vi "HTRB Main.vi"() -> ()   [LabVIEW 2017]
uses:
  Controls/(Ctrl) System State.ctl
  Controls/(Ctrl) State_Test Manage.ctl
  <vilib>/Utility/miscctls.llb/LVPointTypeDef.ctl
  Controls/(Ctrl) State_Display Loop.ctl
  Controls/(Ctrl) State_HVPS CMD.ctl
  Controls/(Ctrl) State_Parcing.ctl
  Controls/(Ctrl) State_Chamber.ctl
  Variables/(Var) Get_HVPS_1.vi
  Variables/(Var) Get_HVPS_2.vi
  Variables/(Var) Get_HVPS_3.vi
  Variables/(Var) Chamber.vi
panel:
  out "G3. State":T1
  out "G2. State":T1
  out "G1. State":T1
  out "Pulse":bool
  out "END":bool=TRUE
  out "G3_TEST END?":bool
  out "G2_TEST END?":bool
  out "G1_TEST END?":bool
  out "Exit ?":bool
  out "탭 컨트롤":enum32{"Display", "Manual Mode", "State"}(tab)
  in  "Start Delay":dbl format="%<%H:%M:%S>t"
  out "G2. Operating Voltage":dbl caption="Operating Voltage" format="%.1f    V"
  in  "G2. Start Delay":dbl caption="Start Delay" format="%<%H:%M:%S>t"
  in  "G1. Start Delay":dbl caption="Start Delay" format="%<%H:%M:%S>t"
  in  "Group3. Info":string
  in  "Group2. Info":string
  in  "Group1. Info":string
  in  "Chamber":bool
  out "G3. Delay":dbl format="%<%H:%M:%S>t"
  out "G2. Delay":dbl format="%<%H:%M:%S>t"
  out "G1. Delay":dbl format="%<%H:%M:%S>t"
  out "G1. Current Graph":cluster{"G1. Current Limit ":dbl, "G1. mA":dbl}(graph)
  out "G1. Voltage Graph":dbl(graph)
  in  "Target Temp":u16 format="%d ℃"
  out "G3. Time":dbl format="%<%H:%M:%S>t"
  in  "G3. Target Time":dbl=460800.0 format="%<%H>t 시간"
  out "G2. Time":dbl format="%<%H:%M:%S>t"
  in  "G2. Target Time":dbl=460800.0 format="%<%H>t 시간"
  out "G1. Time":dbl format="%<%H:%M:%S>t"
  in  "G1. Target Time":dbl=460800.0 format="%<%H>t 시간"
  out "Chamber Temp":dbl format="%.2f ℃"
  out "G3. Current Graph":cluster{"G1. Current Limit ":dbl, "G1. mA":dbl}(graph)
  out "G3. Voltage Graph":dbl(graph)
  out "G2. Current Graph":cluster{"G1. Current Limit ":dbl, "G1. mA":dbl}(graph)
  out "G2. Voltage Graph":dbl(graph)
  in  "Data Save Path":path=path "D:/Raw"
  in  "G3. Stop Butten":bool
  in  "G3. Start Butten":bool
  in  "G2. Stop Butten":bool
  in  "G2. Start Butten":bool
  in  "G1. Stop Butten":bool
  in  "G1. Start Butten":bool
  in  "G2. Taget Voltage":dbl caption="Target Voltage" min=0.0 max=2000.0 format="%.1f V"
  in  "G1. Taget Voltage":dbl caption="Target Voltage" min=0.0 max=2000.0 format="%.1f V"
  in  "G3. Taget Voltage":dbl caption="Target Voltage" min=0.0 max=2000.0 format="%.1f V"
  in  "G3. RB/GB":bool
  out "G3. Test  Status":u16(ring)=1 caption="Test Status"
  out "G3.Comm":bool caption="Communication ="
  out "G3.System":bool caption="System Status ="
  out "G3. Operating Voltage":dbl caption="Operating Voltage" format="%.1f    V"
  out "G3. Leakage Current":dbl caption="Leakage Current" format="%.2f mA"
  in  "G3. Current Limit":dbl caption="Current Limit" format="%.1f mA"
  out "G3. Layout":bool
  in  "G2. RB/GB":bool
  out "G2. Test  Status":u16(ring)=1 caption="Test Status"
  out "G2.Comm":bool caption="Communication ="
  out "G2.System":bool caption="System Status ="
  out "G2. Leakage Current":dbl caption="Leakage Current" format="%.2f mA"
  in  "G2. Current Limit":dbl caption="Current Limit" format="%.1f mA"
  out "G2. Layout":bool
  in  "G1. RB/GB":bool
  out "G1.Comm":bool caption="Communication ="
  out "G1.System":bool caption="System Status ="
  out "G1. Test  Status":u16(ring)=1 caption="Test Status"
  out "G1. Operating Voltage":dbl caption="Operating Voltage" format="%.1f    V"
  out "G1. Leakage Current":dbl caption="Leakage Current" format="%.2f mA"
  in  "G1. Current Limit":dbl caption="Current Limit" format="%.1f mA"
  out "G1. Layout":bool
  out "G1_Disable":bool=TRUE
  out "G3_Disable":bool=TRUE
  out "G2_Disable":bool=TRUE
  out "Data Filename":path
  in  "Exit":bool
  out "G3.Manual_Get mA":dbl format="%3.1f mA"
  out "G3.Manual_Get V":dbl format="%.1f V"
  in  "Group.3 Manual":T2 {"Set mA" items=["0mA"=0, "5mA"=5, "10mA"=10, "15mA"=15, "20mA"=20, "50mA"=50, "70mA"=70, "100mA"=100, "150mA"=150]; "Set V" items=["0V"=0, "10V"=10, "100V"=100, "300V"=300, "500V"=500, "700V"=700, "1000V"=1000, "1500V"=1500]}
  out "G2.Manual_Get mA":dbl format="%3.1f mA"
  out "G2.Manual_Get V":dbl format="%.1f V"
  in  "Group.2 Manual":T2 {"Set mA" items=["0mA"=0, "5mA"=5, "10mA"=10, "15mA"=15, "20mA"=20, "50mA"=50, "70mA"=70, "100mA"=100, "150mA"=150]; "Set V" items=["0V"=0, "10V"=10, "100V"=100, "300V"=300, "500V"=500, "700V"=700, "1000V"=1000, "1500V"=1500]}
  out "G1.Manual_Get mA":dbl format="%3.1f mA"
  out "G1.Manual_Get V":dbl format="%.1f V"
  in  "Group.1 Manual":T2 {"Set mA" items=["0mA"=0, "5mA"=5, "10mA"=10, "15mA"=15, "20mA"=20, "50mA"=50, "70mA"=70, "100mA"=100, "150mA"=150]; "Set V" items=["0V"=0, "10V"=10, "100V"=100, "300V"=300, "500V"=500, "700V"=700, "1000V"=1000, "1500V"=1500]}
  out "G1 System State":T3
  out "G2 System State":T3
  out "G3 System State":T3
  out "error out":errorcluster
  in  "error in (no error)":errorcluster
  in  "Radio_TAB":enum32{"Home", "Manual Mode"}(radio)
  # "ON"
  # "OFF"
  # "High Temperature Reverse Bias Tester"
  # "Software Version 0.0.1"
  # "Group 1"
  # "/"
  # "Group 2"
  # "/"
  # "Group 3"
  # "/"
  # "Group.3 Manual"
  # "Group.2 Manual"
  # "Group.1 Manual"
  # "Group.1 System State"
  # "Voltage Mode On"
  # "Current Mode On"
  # "HV On"
  # "Regulator Error"
  # "Local Mode"
  # "System Fault"
  # "Adjustable Overload Fault"
  # "Over Temperature"
  # "Arc Fault"
  # "Over Power"
  # "Over Current"
  # "Over Voltage Fault"
  # "HV Inhibited"
  # "Interlock open"
  # "Group.2 System State"
  # "Voltage Mode On"
  # "Current Mode On"
  # "HV On"
  # "Regulator Error"
  # "Local Mode"
  # "System Fault"
  # "Adjustable Overload Fault"
  # "Over Temperature"
  # "Arc Fault"
  # "Over Power"
  # "Over Current"
  # "Over Voltage Fault"
  # "HV Inhibited"
  # "Interlock open"
  # "Group.3 System State"
  # "Voltage Mode On"
  # "Current Mode On"
  # "HV On"
  # "Regulator Error"
  # "Local Mode"
  # "System Fault"
  # "Adjustable Overload Fault"
  # "Over Temperature"
  # "Arc Fault"
  # "Over Power"
  # "Over Current"
  # "Over Voltage Fault"
  # "HV Inhibited"
  # "Interlock open"
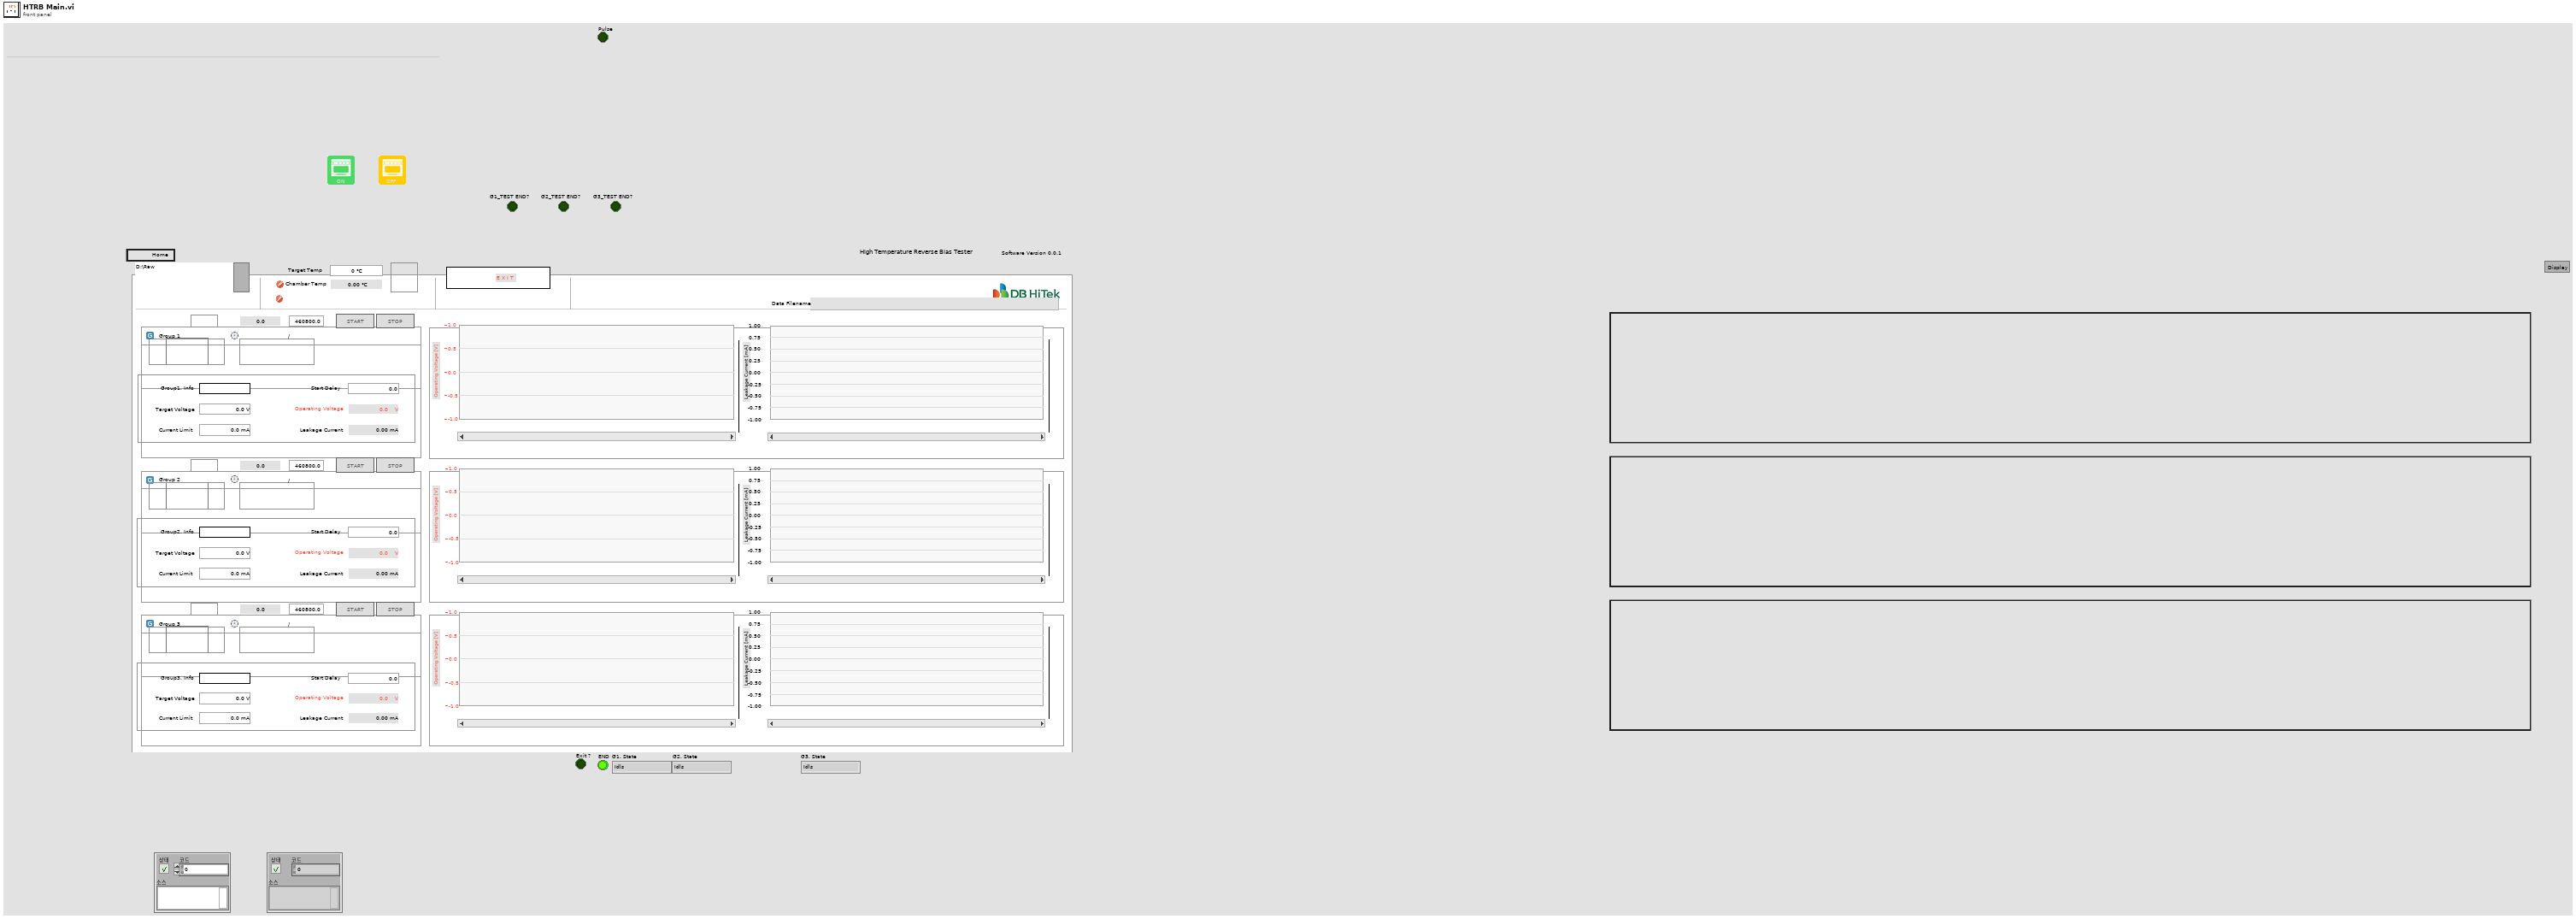
[diagram p1: front panel]
types:
  T1 = typedef "(Ctrl) State_Test Manage.ctl" = enum16{"Idls", "Run Init", "Run", "Rising", "Falling", "Quick Falling", "Close"}
  T2 = cluster{"Bool_HV ON":bool, "Bool_HV OFF":bool, "Bool_Set V":bool, "Bool_Set mA":bool, "Bool_Get V":bool, "Bool_Get mA":bool, "Set V":u16, "Set mA":u16}
  T3 = typedef "(Ctrl) System State.ctl" = cluster{"Interlock open":bool, "HV Inhibited":bool, "Over Voltage Fault":bool, "Over Current":bool, "Over Power":bool, "Regulator Error":bool, "Arc Fault":bool, "Over Temperature":bool, "Adjustable Overload Fault":bool, "System Fault":bool, "Remote Mode":bool, "HV On":bool, "Current Mode On":bool, "Voltage Mode On":bool}
  T4 = typedef "(Ctrl) State_Display Loop.ctl" = enum16{"Init", "Idls", "Run Init", "Run", "Stop", "Close"}
  T5 = typedef "LVPointTypeDef.ctl" = cluster{"Horizontal":i16, "Vertical":i16}
  T6 = typedef "(Ctrl) State_HVPS CMD.ctl" = enum16{"Open", "Rx : V", "Rx : mA", "Rx : State", "Rx : ADC", "Tx : Set V", "Tx : Set mA", "Tx : ON", "Tx : OFF", "Close"}
  T7 = enum8{"Enabled", "Disabled", "Disabled and Grayed Out"}
  T8 = typedef "(Ctrl) State_Chamber.ctl" = enum16{"Open", "Rx : Temp", "Rx : Target Temp", "Rx : State", "Tx : ON-OFF", "Tx : Target Temp", "Tx : Time Set", "Close"}
  T9 = enum16{"G1. Reset", "G2. Reset", "G3. Reset", "G1. Save", "G2. Save", "G3. Save", "G1. Load", "G2. Load", "G3. Load"}
  T10 = cluster{"G1. Current Limit ":dbl, "G1. mA":dbl}[]
  T11 = typedef "(Ctrl) State_Parcing.ctl" = enum16{"Default", "Set V", "Set mA", "Get V", "Get mA", "Get ADC"}
  T12 = enum32{"invalid app kind", "Development System", "Run Time System", "Student Edition", "Embedded LabVIEW", "Evaluation", "Custom"}
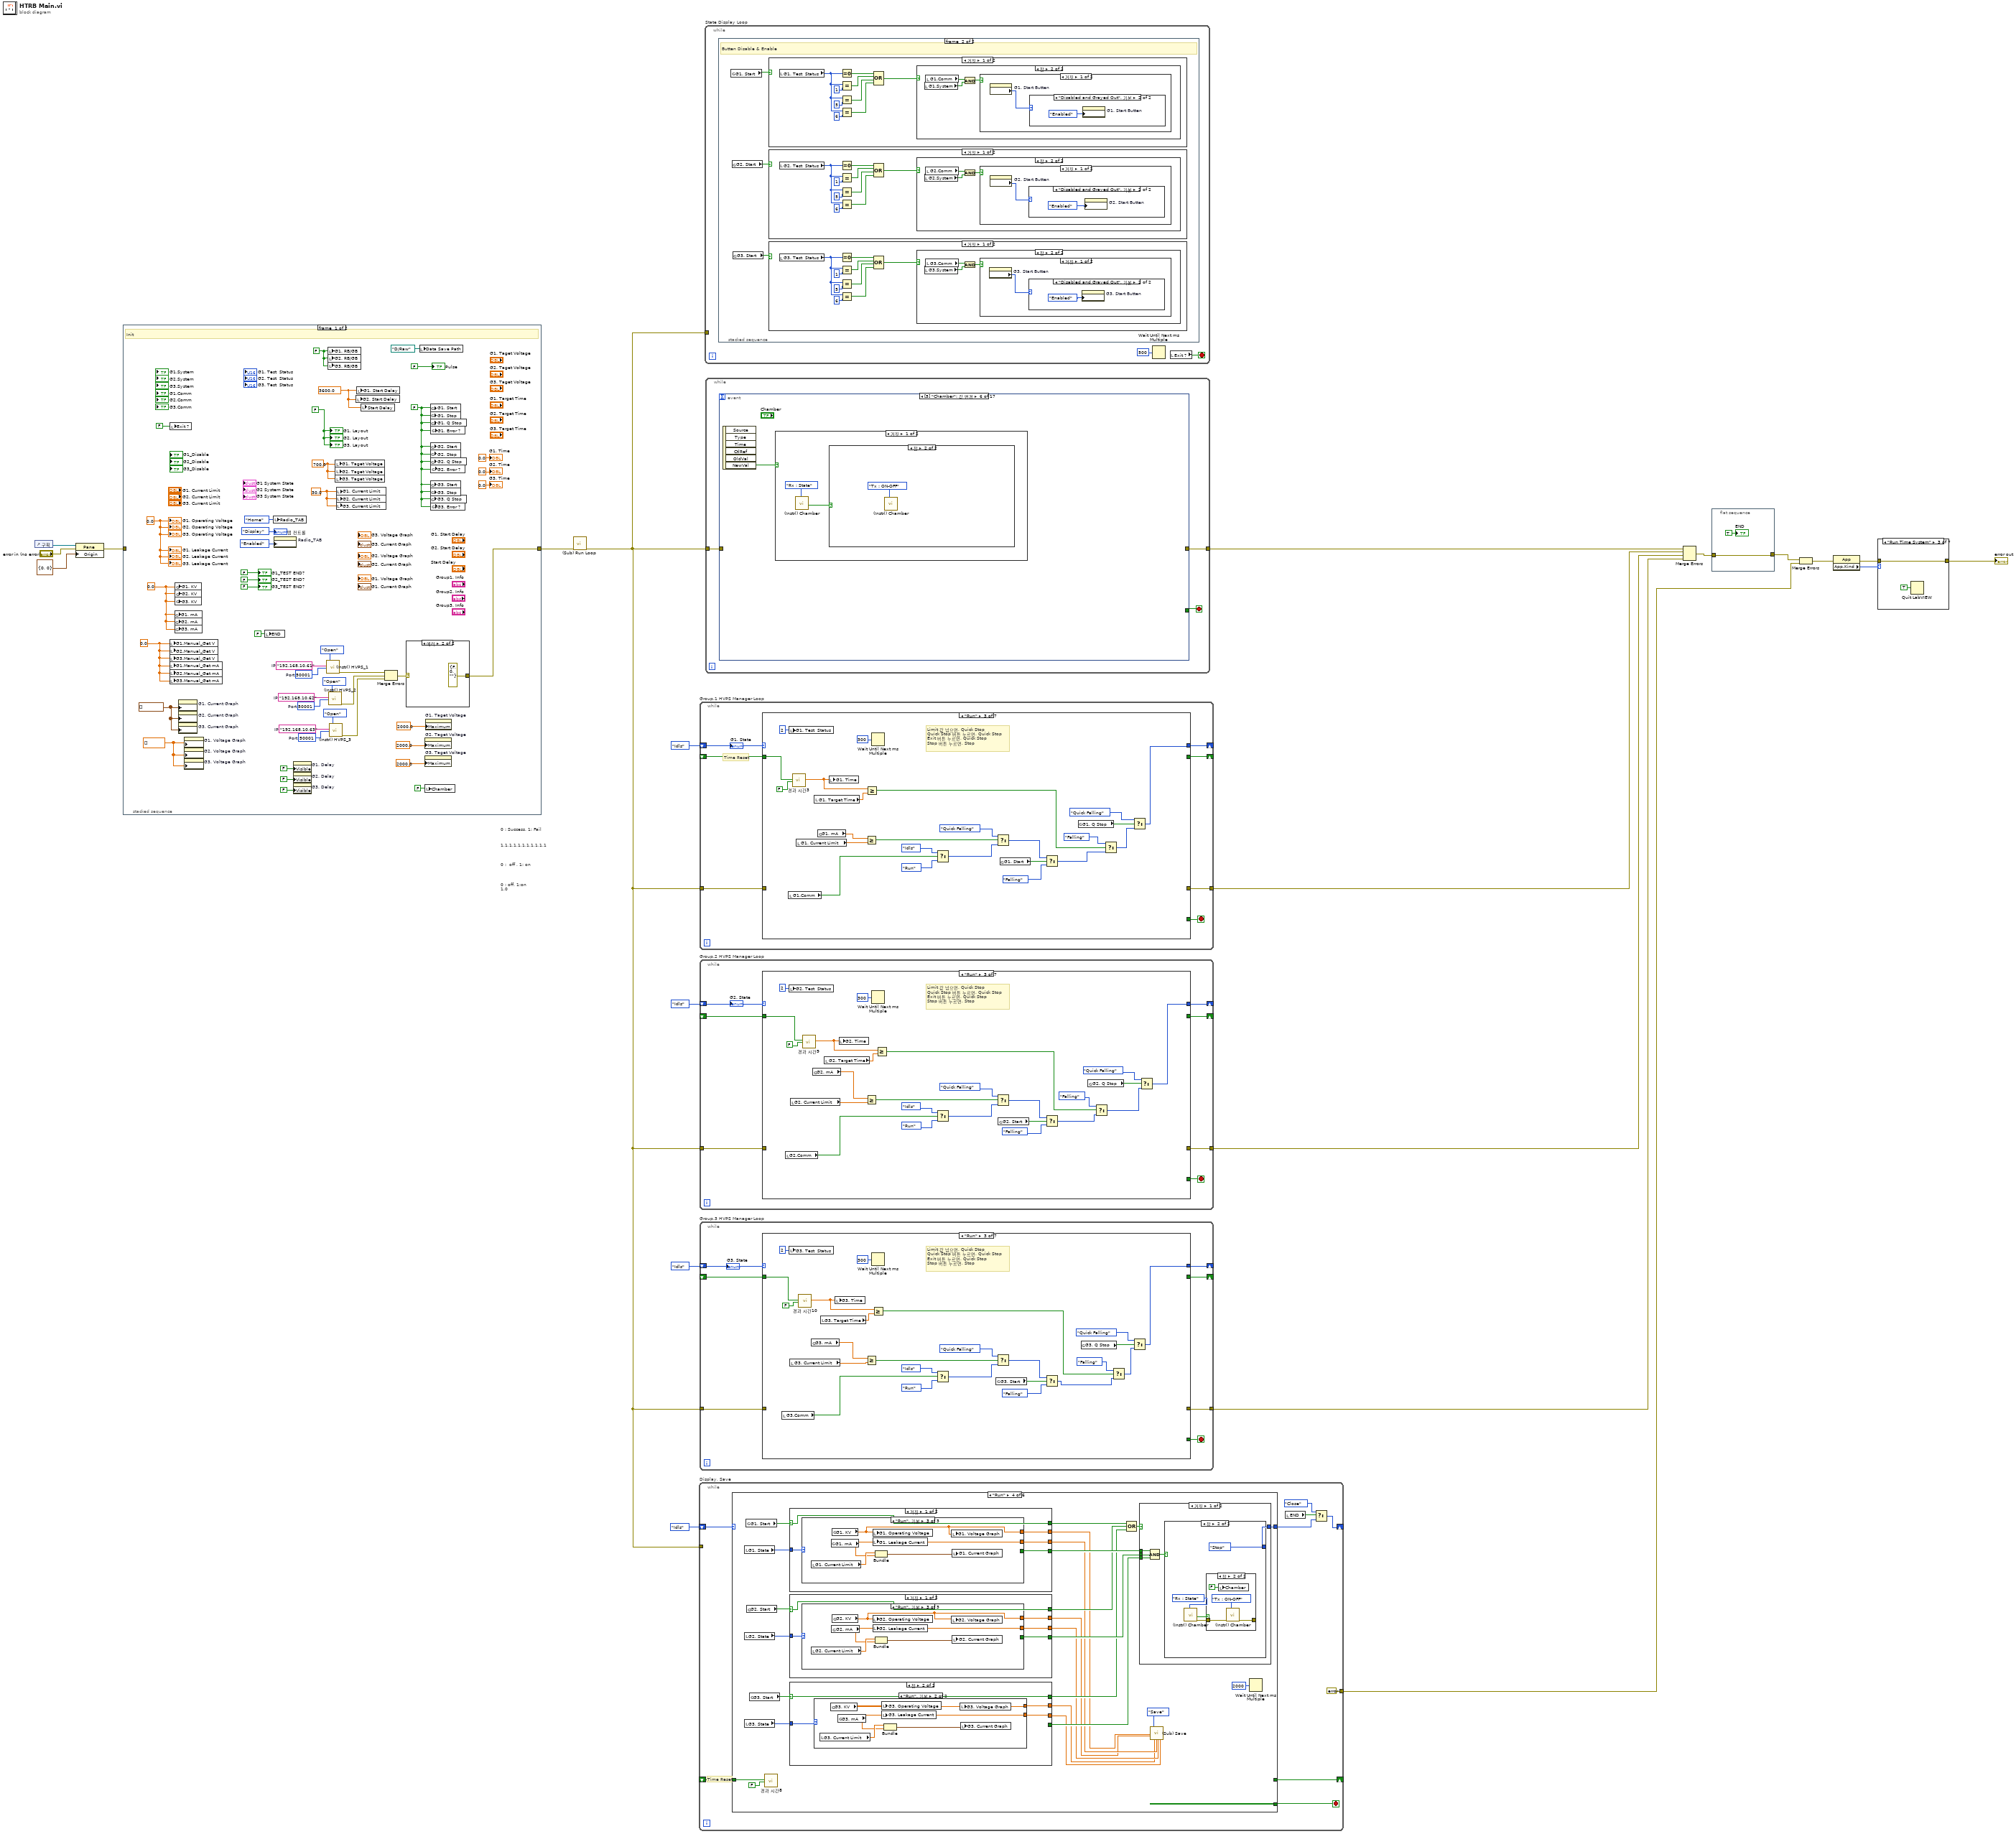
[diagram p0: block diagram]
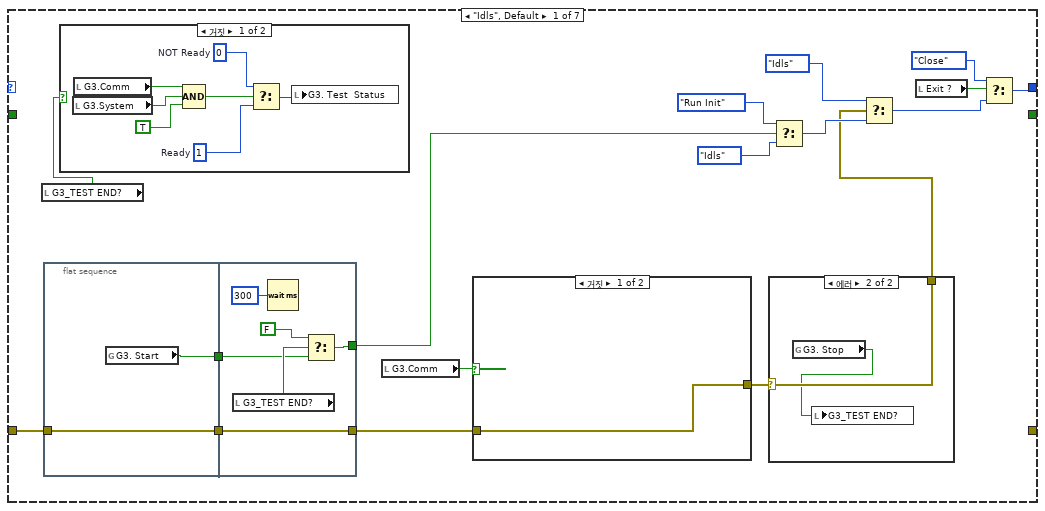
[diagram p2: hidden frame]
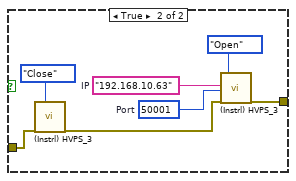
[diagram p3: hidden frame]
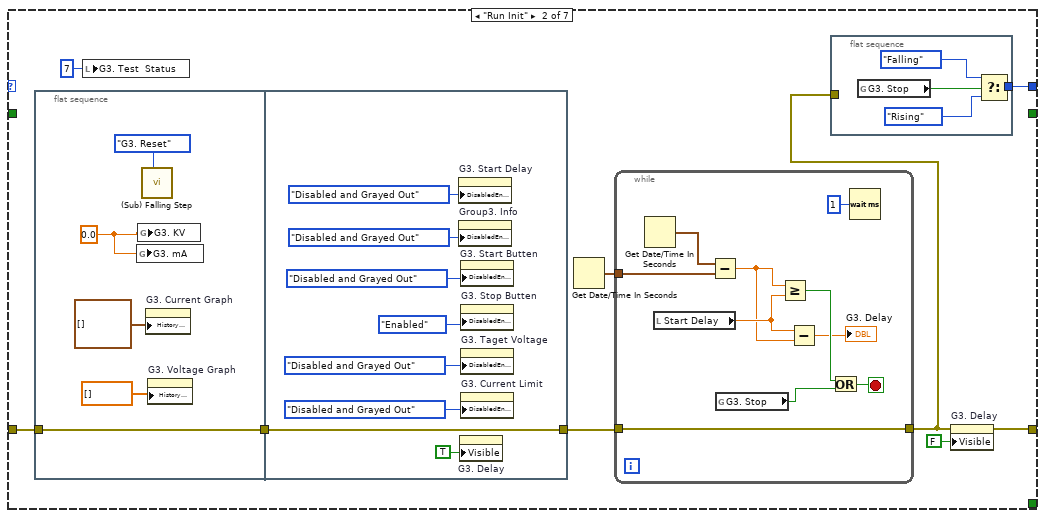
[diagram p6: hidden frame]
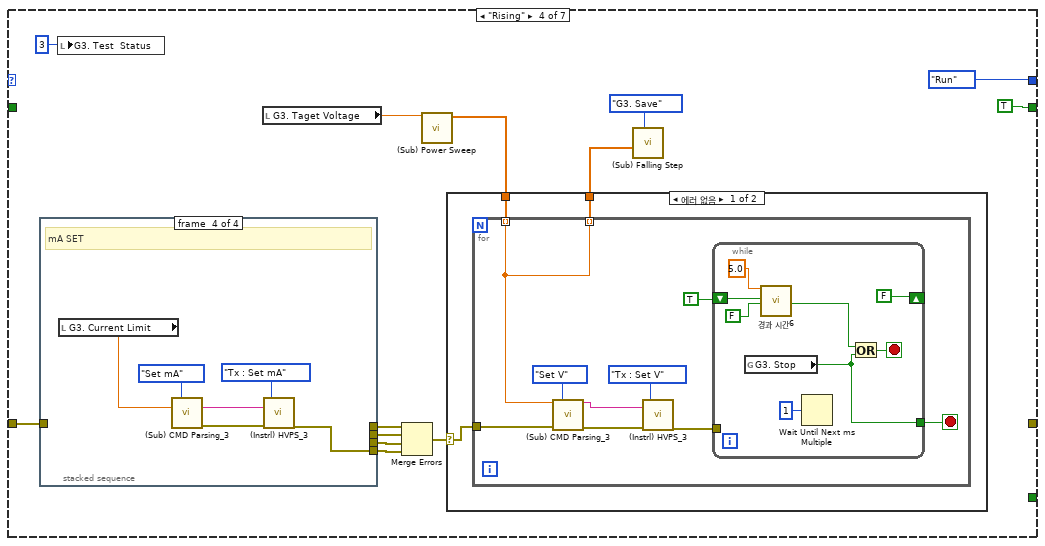
[diagram p7: hidden frame]
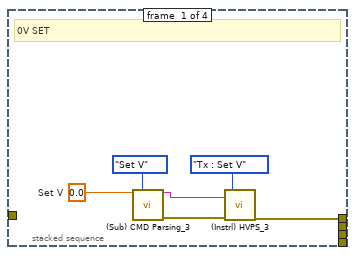
[diagram p9: hidden frame]
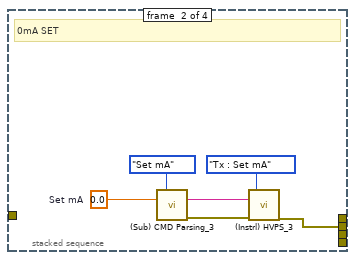
[diagram p10: hidden frame]
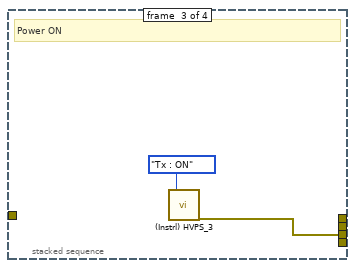
[diagram p11: hidden frame]
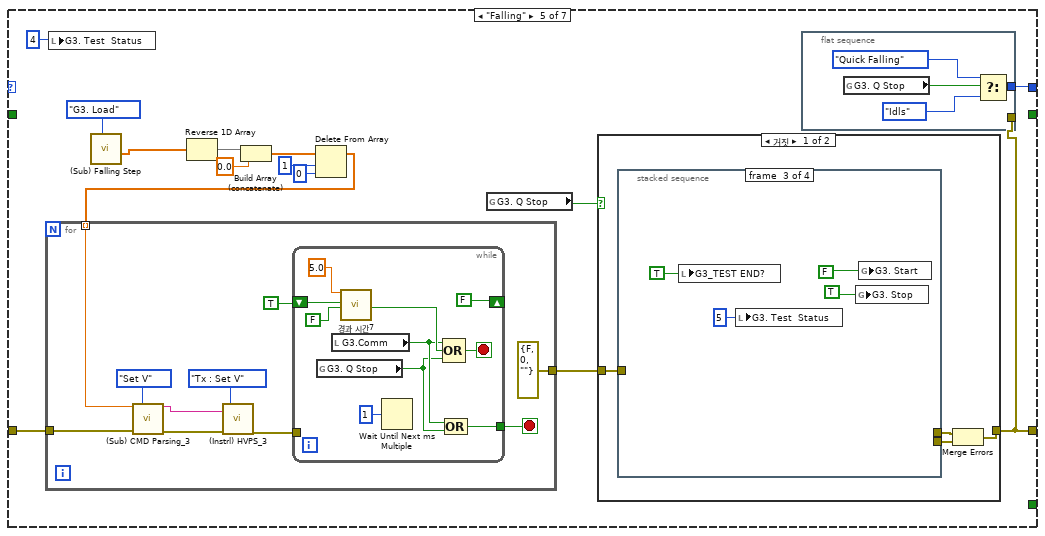
[diagram p12: hidden frame]
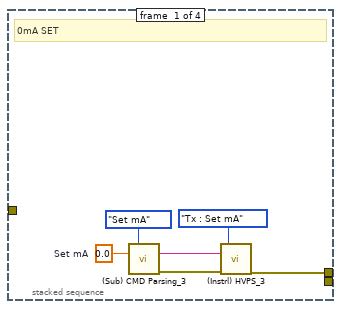
[diagram p13: hidden frame]
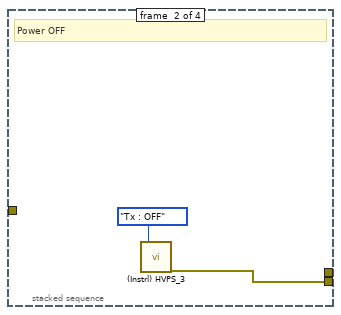
[diagram p14: hidden frame]
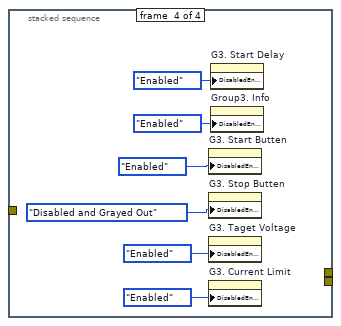
[diagram p15: hidden frame]
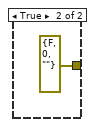
[diagram p16: hidden frame]
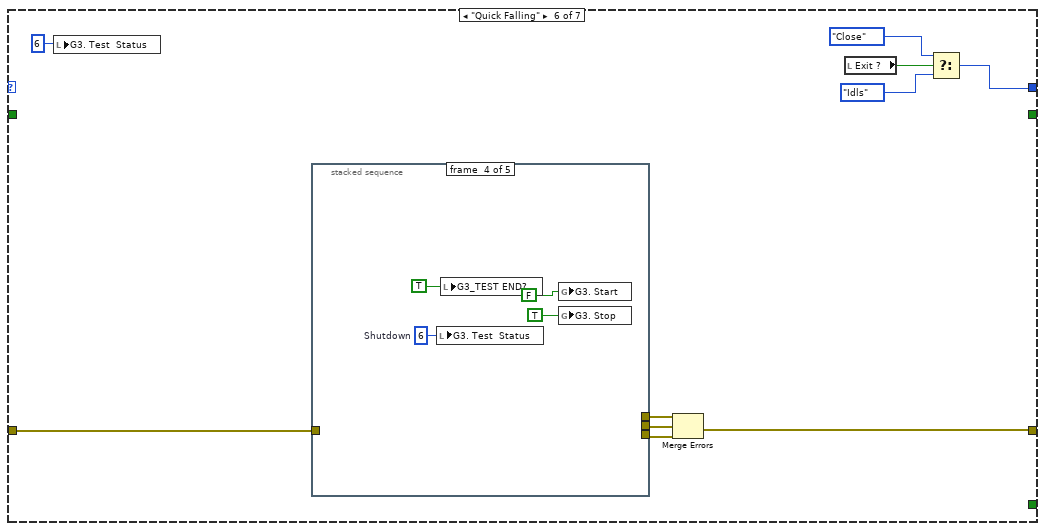
[diagram p17: hidden frame]
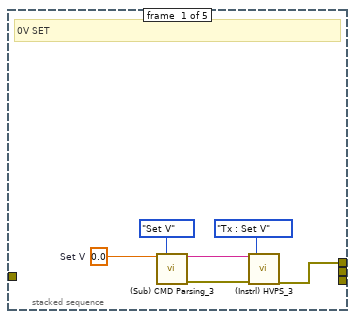
[diagram p18: hidden frame]
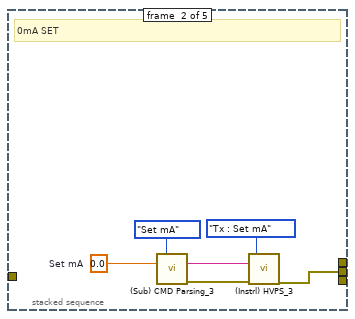
[diagram p19: hidden frame]
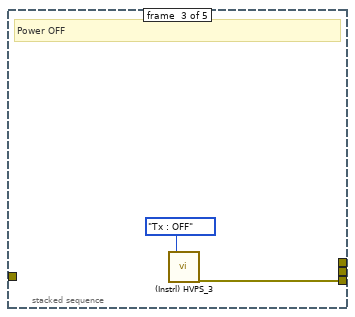
[diagram p20: hidden frame]
diagram:
  # "0 : off, 1:on\n1,0"
  # "0 :  off , 1: on"
  # "1,1,1,1,1,1,1,1,1,1,1"
  # "0 : Success, 1: Fail"
  n1 = control-ref of="구획"() -> (w15:refnum<vi>)
  n2 = property class="Pane"(reference=w15, error in="error in (no error)", "Origin"=T5 {"Horizontal"=0, "Vertical"=0} ("원점")) -> (error out=w12:errorcluster)  [unwired: 1 out]
  n3 = stacked-sequence {
    tunnel: w12 -> [_ _]
    tunnel: [w47 _] -> w2
    frame #0 {
      w27 = 3600.0
      w23 = FALSE
      w39 = FALSE
      w42 = 30.0
      w43 = 700.0
      w40 = FALSE
      w52 = u16 50001  # Port
      w53 = "192.168.10.63"  # IP
      w55 = u16 50001  # Port
      w56 = "192.168.10.62"  # IP
      w58 = u16 50001  # Port
      w59 = "192.168.10.61"  # IP
      w65 = 0.0 ("G1.Manual_Get V")
      w64 = 0.0 ("G1. Current Limit")
      w22 = 0.0 ("G1. KV")
      w38 = cluster{"Current Limit":dbl, "Current":dbl}[] [] ("히스토리 데이터")
      w37 = dbl[] [] ("히스토리 데이터")
      # "Init"
      n4 = local write "G1.Manual_Get V"(w65) -> ()
      n5 = local write "G2.Manual_Get V"(w65) -> ()
      n6 = local write "G3.Manual_Get V"(w65) -> ()
      n7 = local write "G1.Manual_Get mA"(w65) -> ()
      n8 = local write "G2.Manual_Get mA"(w65) -> ()
      n9 = local write "G3.Manual_Get mA"(w65) -> ()
      n10 = local write "Exit ?"(FALSE ("Exit ?")) -> ()
      n11 = global write "(Var) Get_HVPS_1.vi" "G1. mA"(w22) -> ()
      n12 = global write "(Var) Get_HVPS_2.vi" "G2. mA"(w22) -> ()
      n13 = global write "(Var) Get_HVPS_3.vi" "G3. mA"(w22) -> ()
      n14 = global write "(Var) Get_HVPS_1.vi" "G1. KV"(w22) -> ()
      n15 = global write "(Var) Get_HVPS_2.vi" "G2. KV"(w22) -> ()
      n16 = global write "(Var) Get_HVPS_3.vi" "G3. KV"(w22) -> ()
      n17 = property on="G1. Current Graph" class="WFChart (엄격한)"("History Data"=w38) -> ()  [unwired: 2 in, 2 out]
      n18 = property on="G2. Current Graph" class="WFChart (엄격한)"("History Data"=w38) -> ()  [unwired: 2 in, 2 out]
      n19 = property on="G3. Current Graph" class="WFChart (엄격한)"("History Data"=w38) -> ()  [unwired: 2 in, 2 out]
      n20 = property on="G1. Voltage Graph" class="WFChart (엄격한)"("History Data"=w37) -> ()  [unwired: 2 in, 2 out]
      n21 = property on="G2. Voltage Graph" class="WFChart (엄격한)"("History Data"=w37) -> ()  [unwired: 2 in, 2 out]
      n22 = property on="G3. Voltage Graph" class="WFChart (엄격한)"("History Data"=w37) -> ()  [unwired: 2 in, 2 out]
      n23 = local write "END"(FALSE ("END")) -> ()
      n24 = local write "Radio_TAB"(enum32{"Home", "Manual Mode"}."Home" ("Radio_TAB")) -> ()
      n25 = property on="Radio_TAB" class="RadioBtnsControl (엄격한)"("DisabledEnum"=T7."Enabled" ("비활성화")) -> ()  [unwired: 2 in, 2 out]
      n26 = property on="G1. Delay" class="DigNum (엄격한)"("Visible"=FALSE ("보이기")) -> ()  [unwired: 2 in, 2 out]
      n27 = property on="G2. Delay" class="DigNum (엄격한)"("Visible"=FALSE ("보이기")) -> ()  [unwired: 2 in, 2 out]
      n28 = property on="G3. Delay" class="DigNum (엄격한)"("Visible"=FALSE ("보이기")) -> ()  [unwired: 2 in, 2 out]
      n29 = call "(Instrl) HVPS_1.vi"("IP"=w59, "Port"=w58, "CMD"=(Ctrl)_State_HVPS_CMD."Open" ("State")) -> ("error out"=w51:errorcluster)  [unwired: 11 in, 5 out]
      n30 = local write "G1. RB/GB"(w40) -> ()
      n31 = local write "G2. RB/GB"(w40) -> ()
      n32 = local write "G3. RB/GB"(w40) -> ()
      n33 = call "(Instrl) HVPS_2.vi"("IP"=w56, "Port"=w55, "CMD"=(Ctrl)_State_HVPS_CMD."Open" ("State")) -> ("error out"=w50:errorcluster)  [unwired: 11 in, 5 out]
      n34 = call "(Instrl) HVPS_3.vi"("IP"=w53, "Port"=w52, "CMD"=(Ctrl)_State_HVPS_CMD."Open" ("State")) -> ("error out"=w49:errorcluster)  [unwired: 11 in, 5 out]
      n35 = local write "G1. Taget Voltage"(w43) -> ()
      n36 = local write "G2. Taget Voltage"(w43) -> ()
      n37 = local write "G3. Taget Voltage"(w43) -> ()
      n38 = local write "G1. Current Limit"(w42) -> ()
      n39 = local write "G2. Current Limit"(w42) -> ()
      n40 = local write "G3. Current Limit"(w42) -> ()
      n41 = local write "G2. Start Delay"(w27) -> ()
      n42 = local write "G1. Start Delay"(w27) -> ()
      n43 = local write "Start Delay"(w27) -> ()
      n44 = Merge Errors(w51, w50, w49) -> (w48:errorcluster)
      n45 = case shown="에러" w48 {
        selector: w48 -> [w67 _]
        tunnel: [w67 errorcluster {"status"=FALSE, "code"=0, "source"=""} ("에러 상수")] -> w47
        frame No Error {
        }
        frame Error {
        }
      }
      n46 = local write "Data Save Path"(path "D:/Raw" ("Data Save Path")) -> ()
      n47 = property on="G2. Taget Voltage" class="DigNum (엄격한)"("Maximum"=2000.0 ("데이터 입력 제한:최대")) -> ()  [unwired: 2 in, 2 out]
      n48 = property on="G3. Taget Voltage" class="DigNum (엄격한)"("Maximum"=2000.0 ("데이터 입력 제한:최대")) -> ()  [unwired: 2 in, 2 out]
      n49 = local write "Chamber"(FALSE ("Chamber")) -> ()
      n50 = property on="G1. Taget Voltage" class="DigNum (엄격한)"("Maximum"=2000.0 ("데이터 입력 제한:최대")) -> ()  [unwired: 2 in, 2 out]
      n51 = global write "(Var) Get_HVPS_1.vi" "G1. Start"(w23) -> ()
      n52 = global write "(Var) Get_HVPS_1.vi" "G1. Stop"(w23) -> ()
      n53 = global write "(Var) Get_HVPS_1.vi" "G1. Q Stop"(w23) -> ()
      n54 = global write "(Var) Get_HVPS_2.vi" "G2. Start"(w23) -> ()
      n55 = global write "(Var) Get_HVPS_2.vi" "G2. Stop"(w23) -> ()
      n56 = global write "(Var) Get_HVPS_2.vi" "G2. Q Stop"(w23) -> ()
      n57 = global write "(Var) Get_HVPS_3.vi" "G3. Start"(w23) -> ()
      n58 = global write "(Var) Get_HVPS_3.vi" "G3. Stop"(w23) -> ()
      n59 = global write "(Var) Get_HVPS_3.vi" "G3. Q Stop"(w23) -> ()
      n60 = global write "(Var) Get_HVPS_1.vi" "G1. Error ?"(w23) -> ()
      n61 = global write "(Var) Get_HVPS_2.vi" "G2. Error ?"(w23) -> ()
      n62 = global write "(Var) Get_HVPS_3.vi" "G3. Error ?"(w23) -> ()
      "G1. Leakage Current" <- w64
      "G1. Operating Voltage" <- w64
      "G2. Leakage Current" <- w64
      "G2. Operating Voltage" <- w64
      "G3. Leakage Current" <- w64
      "G3. Operating Voltage" <- w64
      "탭 컨트롤" <- enum32{"Display", "Manual Mode", "State"}."Display" ("탭 컨트롤")
      "G1_TEST END?" <- FALSE ("G1_TEST END?")
      "G2_TEST END?" <- FALSE ("G1_TEST END?")
      "G3_TEST END?" <- FALSE ("G1_TEST END?")
      "G1. Layout" <- w39
      "G3. Layout" <- w39
      "G2. Layout" <- w39
      "Pulse" <- FALSE
      "G1. Time" <- 0.0 ("G1. Time")
      "G2. Time" <- 0.0 ("G2. Time")
      "G3. Time" <- 0.0 ("G3. Time")
    }
    frame #1 {
      n63 = property on="G2. Start Delay" class="DigNum (엄격한)"("DisabledEnum"=T7."Enabled" ("비활성화")) -> ()  [unwired: 2 in, 2 out]
      n64 = property on="Group2. Info" class="Str"("DisabledEnum"=T7."Enabled" ("비활성화")) -> ()  [unwired: 2 in, 2 out]
      n65 = property on="G2. Start Butten" class="Bool"("DisabledEnum"=T7."Enabled" ("비활성화")) -> ()  [unwired: 2 in, 2 out]
      n66 = property on="G2. Stop Butten" class="Bool"("DisabledEnum"=T7."Disabled and Grayed Out" ("비활성화")) -> ()  [unwired: 2 in, 2 out]
      n67 = property on="G2. Taget Voltage" class="DigNum (엄격한)"("DisabledEnum"=T7."Enabled" ("비활성화")) -> ()  [unwired: 2 in, 2 out]
      n68 = property on="G2. Current Limit" class="DigNum (엄격한)"("DisabledEnum"=T7."Enabled" ("비활성화")) -> ()  [unwired: 2 in, 2 out]
      n69 = property on="G3. Start Butten" class="Bool"("DisabledEnum"=T7."Enabled" ("비활성화")) -> ()  [unwired: 2 in, 2 out]
      n70 = property on="G3. Stop Butten" class="Bool"("DisabledEnum"=T7."Disabled and Grayed Out" ("비활성화")) -> ()  [unwired: 2 in, 2 out]
      n71 = property on="G3. Taget Voltage" class="DigNum (엄격한)"("DisabledEnum"=T7."Enabled" ("비활성화")) -> ()  [unwired: 2 in, 2 out]
      n72 = property on="G3. Current Limit" class="DigNum (엄격한)"("DisabledEnum"=T7."Enabled" ("비활성화")) -> ()  [unwired: 2 in, 2 out]
      n73 = property on="G1. Start Butten" class="Bool"("DisabledEnum"=T7."Enabled" ("비활성화")) -> ()  [unwired: 2 in, 2 out]
      n74 = property on="G1. Stop Butten" class="Bool"("DisabledEnum"=T7."Disabled and Grayed Out" ("비활성화")) -> ()  [unwired: 2 in, 2 out]
      n75 = property on="G1. Taget Voltage" class="DigNum (엄격한)"("DisabledEnum"=T7."Enabled" ("비활성화")) -> ()  [unwired: 2 in, 2 out]
      n76 = property on="Group1. Info" class="Str"("DisabledEnum"=T7."Enabled" ("비활성화")) -> ()  [unwired: 2 in, 2 out]
      n77 = property on="Start Delay" class="DigNum (엄격한)"("DisabledEnum"=T7."Enabled" ("비활성화")) -> ()  [unwired: 2 in, 2 out]
      n78 = property on="G1. Start Delay" class="DigNum (엄격한)"("DisabledEnum"=T7."Enabled" ("비활성화")) -> ()  [unwired: 2 in, 2 out]
      n79 = property on="G1. Current Limit" class="DigNum (엄격한)"("DisabledEnum"=T7."Enabled" ("비활성화")) -> ()  [unwired: 2 in, 2 out]
      n80 = property on="Group3. Info" class="Str"("DisabledEnum"=T7."Enabled" ("비활성화")) -> ()  [unwired: 2 in, 2 out]
    }
  }
  n81 = call "(Sub) Run Loop.vi"("error in (no error)"=w2) -> ("error out"=w1:errorcluster)  [unwired: 10 in]
  n82 = while "Display, Save" {
    tunnel: w1 -> [_]
    tunnel: [errorcluster {"status"=FALSE, "code"=0, "source"=""} ("에러 상수")] -> w10
    shift-right: [w92] -> _
    shift-left: _ -> [w93]
    shift-right: [w90] -> _
    shift-left: (Ctrl)_State_Display_Loop."Idls" ("열거형") -> [w91]
    stop <- w95 stop-if-true
    # "Time Reset"
    n83 = case shown="\"Run\"" w91 {
      tunnel: [_ _ _ _ _ TRUE] -> w95
      tunnel: w93 -> [_ _ _ w150 _ _]
      tunnel: [TRUE _ TRUE _ _ _] -> w92
      tunnel: [_ w100 (Ctrl)_State_Display_Loop."Run" ("열거형") w148 (Ctrl)_State_Display_Loop."Idls" ("열거형") (Ctrl)_State_Display_Loop."Close" ("열거형")] -> w87
      frame "Init", Default {
      }
      frame "Idls" {
        n84 = Wait (ms)(milliseconds to wait=u32 300 ("ms 배수")) -> ()  [unwired: 1 out]
        n85 = global read "(Var) Get_HVPS_2.vi" "G2. Start"() -> (w98:bool)
        n86 = global read "(Var) Get_HVPS_3.vi" "G3. Start"() -> (w97:bool)
        n87 = global read "(Var) Get_HVPS_1.vi" "G1. Start"() -> (w99:bool)
        n88 = Compound Arithmetic op=OR ("복합 연산")(w99, w98, w97) -> (w103:bool)
        n89 = Select(t=(Ctrl)_State_Display_Loop."Run Init" ("열거형"), s=w103, f=(Ctrl)_State_Display_Loop."Idls" ("열거형")) -> (s? t:f=w100:T4)
      }
      frame "Run Init" {
        n90 = local read "G1. Taget Voltage"() -> (w111:dbl)
        n91 = local read "G2. Taget Voltage"() -> (w110:dbl)
        n92 = local read "G3. Taget Voltage"() -> (w109:dbl)
        n93 = local read "G1. Current Limit"() -> (w114:dbl)
        n94 = local read "G2. Current Limit"() -> (w113:dbl)
        n95 = local read "G3. Current Limit"() -> (w112:dbl)
        n96 = local read "Group1. Info"() -> (w107:string)
        n97 = local read "Group2. Info"() -> (w106:string)
        n98 = local read "Group3. Info"() -> (w105:string)
        n99 = Build Array(w114, w113, w112, w111, w110, w109) -> (w108:dbl[])
        n100 = flat-sequence {
          tunnel: "Data Save Path" -> [w122]
          tunnel: w108 -> [w120]
          tunnel: [w121] -> w117
          tunnel: [w120] -> w116
          tunnel: w107 -> [_]
          tunnel: w106 -> [_]
          tunnel: w105 -> [_]
          tunnel: w117 -> [w126]
          tunnel: w116 -> [w125]
          frame #0 {
            n101 = call "(Sub) Save.vi"("IN Path"=w122, "State"=enum16{"Open", "Header Make", "Save", "Close"}."Open") -> ("Save Path"=→"Data Filename":path, "error out"=w121:errorcluster)  [unwired: 16 in]
          }
          frame #1 {
            n102 = call "(Sub) Save.vi"("C Limit / Voltage"=w125, "error in (no error)"=w126, "State"=enum16{"Open", "Header Make", "Save", "Close"}."Header Make") -> ()  [unwired: 15 in, 2 out]
          }
        }
      }
      frame "Run" {
        n103 = local read "G1. State"() -> (w145:T1)
        n104 = local read "G2. State"() -> (w143:T1)
        n105 = local read "G3. State"() -> (w142:T1)
        n106 = global read "(Var) Get_HVPS_1.vi" "G1. Start"() -> (w137:bool)
        n107 = global read "(Var) Get_HVPS_2.vi" "G2. Start"() -> (w136:bool)
        n108 = global read "(Var) Get_HVPS_3.vi" "G3. Start"() -> (w135:bool)
        n109 = call "경과 시간8"("Reset"=w150, "Auto Reset"=FALSE) -> ()  [unwired: 10 in, 8 out]
        n110 = case shown="거짓" w137 {
          selector: w137 -> [w220 w236]
          tunnel: [w222 w235] -> w133
          tunnel: [w221 w234] -> w132
          tunnel: [w220 w236] -> w147
          tunnel: w145 -> [w219 w233]
          tunnel: [w218 _] -> w144
          frame False {
            n111 = case shown="\"Run\", 기본" w219 {
              tunnel: [nan nan w229] -> w222
              tunnel: [nan nan w230] -> w221
              tunnel: [TRUE TRUE _] -> w218
              frame "Idls" {
              }
              frame "Run Init" {
              }
              frame "Run", Default {
                n112 = local read "G1. Current Limit"() -> (w232:dbl)
                n113 = global read "(Var) Get_HVPS_1.vi" "G1. mA"() -> (w230:dbl)
                n114 = global read "(Var) Get_HVPS_1.vi" "G1. KV"() -> (w229:dbl)
                n115 = local write "G1. Operating Voltage"(w229) -> ()
                n116 = local write "G1. Leakage Current"(w230) -> ()
                n117 = Bundle("G1. Current Limit"=w232, "G1. mA"=w230) -> (w231:cluster{"G1. Current Limit ":dbl, "G1. mA":dbl})  [unwired: 1 in]
                n118 = local write "G1. Voltage Graph"(w229) -> ()
                n119 = local write "G1. Current Graph"(w231) -> ()
              }
            }
          }
          frame True {
            n120 = case shown="\"Run\", 기본" w233 {
              tunnel: [nan w240] -> w235
              tunnel: [nan w239] -> w234
              frame "Run Init" {
              }
              frame "Run", Default {
                n121 = local read "G1. Current Limit"() -> (w242:dbl)
                n122 = global read "(Var) Get_HVPS_1.vi" "G1. mA"() -> (w239:dbl)
                n123 = global read "(Var) Get_HVPS_1.vi" "G1. KV"() -> (w240:dbl)
                n124 = local write "G1. Operating Voltage"(w240) -> ()
                n125 = local write "G1. Leakage Current"(w239) -> ()
                n126 = Bundle("G1. Current Limit"=w242, "G1. mA"=w239) -> (w241:cluster{"G1. Current Limit ":dbl, "G1. mA":dbl})  [unwired: 1 in]
                n127 = local write "G1. Voltage Graph"(w240) -> ()
                n128 = local write "G1. Current Graph"(w241) -> ()
              }
            }
          }
        }
        n129 = case shown="거짓" w136 {
          selector: w136 -> [w179 w195]
          tunnel: [w181 w194] -> w131
          tunnel: [w180 w193] -> w130
          tunnel: [w179 w195] -> w141
          tunnel: w143 -> [w178 w192]
          tunnel: [w177 _] -> w140
          frame False {
            n130 = case shown="\"Run\", 기본" w178 {
              tunnel: [nan nan w188] -> w181
              tunnel: [nan nan w189] -> w180
              tunnel: [TRUE TRUE _] -> w177
              frame "Idls" {
              }
              frame "Run Init" {
              }
              frame "Run", Default {
                n131 = local read "G2. Current Limit"() -> (w191:dbl)
                n132 = global read "(Var) Get_HVPS_2.vi" "G2. mA"() -> (w189:dbl)
                n133 = global read "(Var) Get_HVPS_2.vi" "G2. KV"() -> (w188:dbl)
                n134 = local write "G2. Operating Voltage"(w188) -> ()
                n135 = local write "G2. Leakage Current"(w189) -> ()
                n136 = Bundle("G2. Current Limit"=w191, "G2. mA"=w189) -> (w190:cluster{"G2. Current Limit ":dbl, "G2. mA":dbl})  [unwired: 1 in]
                n137 = local write "G2. Voltage Graph"(w188) -> ()
                n138 = local write "G2. Current Graph"(w190) -> ()
              }
            }
          }
          frame True {
            n139 = case shown="\"Run\", 기본" w192 {
              tunnel: [nan w198] -> w194
              tunnel: [nan w199] -> w193
              frame "Run Init" {
              }
              frame "Run", Default {
                n140 = local read "G2. Current Limit"() -> (w201:dbl)
                n141 = global read "(Var) Get_HVPS_2.vi" "G2. mA"() -> (w199:dbl)
                n142 = global read "(Var) Get_HVPS_2.vi" "G2. KV"() -> (w198:dbl)
                n143 = local write "G2. Operating Voltage"(w198) -> ()
                n144 = local write "G2. Leakage Current"(w199) -> ()
                n145 = Bundle("G2. Current Limit"=w201, "G2. mA"=w199) -> (w200:cluster{"G2. Current Limit ":dbl, "G2. mA":dbl})  [unwired: 1 in]
                n146 = local write "G2. Voltage Graph"(w198) -> ()
                n147 = local write "G2. Current Graph"(w200) -> ()
              }
            }
          }
        }
        n148 = case shown="참" w135 {
          selector: w135 -> [w154 w170]
          tunnel: [w156 w169] -> w129
          tunnel: [w155 w168] -> w128
          tunnel: [w154 w170] -> w139
          tunnel: w142 -> [w153 w167]
          tunnel: [w152 _] -> w138
          frame False {
            n149 = case shown="\"Run\", 기본" w153 {
              tunnel: [nan nan w164] -> w156
              tunnel: [nan nan w163] -> w155
              tunnel: [TRUE TRUE _] -> w152
              frame "Idls" {
              }
              frame "Run Init" {
              }
              frame "Run", Default {
                n150 = local read "G3. Current Limit"() -> (w166:dbl)
                n151 = global read "(Var) Get_HVPS_3.vi" "G3. mA"() -> (w163:dbl)
                n152 = global read "(Var) Get_HVPS_3.vi" "G3. KV"() -> (w164:dbl)
                n153 = local write "G3. Operating Voltage"(w164) -> ()
                n154 = local write "G3. Leakage Current"(w163) -> ()
                n155 = Bundle("G3. Current Limit"=w166, "G3. mA"=w163) -> (w165:cluster{"G3. Current Limit ":dbl, "G3. mA":dbl})  [unwired: 1 in]
                n156 = local write "G3. Voltage Graph"(w164) -> ()
                n157 = local write "G3. Current Graph"(w165) -> ()
              }
            }
          }
          frame True {
            n158 = case shown="\"Run\", 기본" w167 {
              tunnel: [nan w174] -> w169
              tunnel: [nan w173] -> w168
              frame "Run Init" {
              }
              frame "Run", Default {
                n159 = local read "G3. Current Limit"() -> (w176:dbl)
                n160 = global read "(Var) Get_HVPS_3.vi" "G3. KV"() -> (w174:dbl)
                n161 = global read "(Var) Get_HVPS_3.vi" "G3. mA"() -> (w173:dbl)
                n162 = local write "G3. Operating Voltage"(w174) -> ()
                n163 = local write "G3. Leakage Current"(w173) -> ()
                n164 = Bundle("G3. Current Limit"=w176, "G3. mA"=w173) -> (w175:cluster{"G3. Current Limit ":dbl, "G3. mA":dbl})  [unwired: 1 in]
                n165 = local write "G3. Voltage Graph"(w174) -> ()
                n166 = local write "G3. Current Graph"(w175) -> ()
              }
            }
          }
        }
        n167 = Compound Arithmetic op=OR ("복합 연산")(w147, w141, w139) -> (w146:bool)
        n168 = case shown="거짓" w146 {
          tunnel: [w206 (Ctrl)_State_Display_Loop."Run" ("열거형")] -> w148
          tunnel: w144 -> [w205 _]
          tunnel: w140 -> [w204 _]
          tunnel: w138 -> [w203 _]
          frame False {
            n169 = Compound Arithmetic op=AND ("복합 연산")(w205, w204, w203) -> (w202:bool)
            n170 = case shown="참" w202 {
              tunnel: [(Ctrl)_State_Display_Loop."Run" ("열거형") (Ctrl)_State_Display_Loop."Stop" ("열거형")] -> w206
              frame False {
              }
              frame True {
                n171 = call "(Instrl) Chamber.vi"("State"=(Ctrl)_State_Chamber."Rx : State") -> ("error out"=w209:errorcluster, "Run ?"=w210:bool)  [unwired: 7 in, 2 out]
                n172 = case shown="참" w210 {
                  tunnel: w209 -> [w212 w216]
                  tunnel: [w212 w214] -> _
                  frame False {
                  }
                  frame True {
                    n173 = local write "Chamber"(FALSE ("Chamber")) -> ()
                    n174 = call "(Instrl) Chamber.vi"("State"=(Ctrl)_State_Chamber."Tx : ON-OFF", "error in (no error)"=w216) -> ("error out"=w214:errorcluster)  [unwired: 6 in, 3 out]
                  }
                }
              }
            }
          }
          frame True {
          }
        }
        n175 = call "(Sub) Save.vi"("G1. V"=w133, "G2. V"=w131, "State"=enum16{"Open", "Header Make", "Save", "Close"}."Save", "G3. V"=w129, "G1. A"=w132, "G2. A"=w130, "G3. A"=w128) -> ()  [unwired: 11 in, 2 out]
        n176 = Wait Until Next ms Multiple(millisecond multiple=u32 2000 ("대기 시간 (ms)")) -> ()  [unwired: 1 out]
      }
      frame "Stop" {
        n177 = property on="Pulse" class="Bool (엄격한)"("Val(Sgnl)"=FALSE ("값(신호)")) -> ()  [unwired: 2 in, 2 out]
      }
      frame "Close" {
      }
    }
    n178 = local read "END"() -> (w89:bool)
    n179 = Select(t=(Ctrl)_State_Display_Loop."Close" ("열거형"), s=w89, f=w87) -> (s? t:f=w90:T4)
  }
  n180 = while "Group.1 HVPS Manager Loop" {
    shift-right: [w252] -> _
    shift-left: (Ctrl)_State_Test_Manage."Idls" ("State") -> [w253]
    tunnel: w1 -> [w249]
    tunnel: [w250] -> w17
    shift-right: [w248] -> _
    shift-left: _ -> [w247]
    stop <- w251 stop-if-true
    # "Time Reset"
    n181 = case shown="\"Run\"" w253 {
      tunnel: [w263 w300 w346 (Ctrl)_State_Test_Manage."Run" ("State") w423 w480 (Ctrl)_State_Test_Manage."Close" ("State")] -> w252
      tunnel: [_ _ _ _ _ _ TRUE] -> w251
      tunnel: w249 -> [w267 w305 _ w369 w425 w482 w507]
      tunnel: [_ w298 _ _ w415 w474 w508] -> w250
      tunnel: [_ _ _ TRUE _ _ _] -> w248
      tunnel: w247 -> [_ _ w342 _ _ _ _]
      frame "Idls", Default {
        n182 = flat-sequence {
          tunnel: w267 -> [w290]
          tunnel: [w289] -> w269
          tunnel: [w290] -> w268
          tunnel: [w296] -> w262
          tunnel: w269 -> [w293]
          tunnel: w268 -> [w296]
          tunnel: [w291] -> w261
          frame #0 {
            n183 = global read "(Var) Get_HVPS_1.vi" "G1. Start"() -> (w289:bool)
          }
          frame #1 {
            n184 = local read "G1_TEST END?"() -> (w294:bool)
            n185 = Wait (ms)(milliseconds to wait=u32 300 ("대기 시간 (ms)")) -> ()  [unwired: 1 out]
            n186 = Select(t=FALSE, s=w294, f=w293) -> (s? t:f=w291:bool)
          }
        }
        n187 = local read "G1_TEST END?"() -> (w256:bool)
        n188 = case shown="거짓" w256 {
          frame False {
            w283 = 1  # Ready
            w284 = 0  # NOT Ready
            n189 = local read "G1.System"() -> (w287:bool)
            n190 = local read "G1.Comm"() -> (w288:bool)
            n191 = Compound Arithmetic op=AND(w288, w287, TRUE) -> (w285:bool)
            n192 = Select(t=w284, s=w285, f=w283) -> (s? t:f=w282:i32)
            n193 = local write "G1. Test  Status"(w282) -> ()
          }
          frame True {
          }
        }
        n194 = local read "G1.Comm"() -> (w254:bool)
        n195 = case shown="참" w254 {
          tunnel: w262 -> [w271 w274]
          tunnel: [w271 w277] -> w255
          frame False {
          }
          frame True {
            w275 = u16 50001  # Port
            w276 = "192.168.10.61"  # IP
            n196 = call "(Instrl) HVPS_1.vi"("error in (no error)"=w274, "CMD"=(Ctrl)_State_HVPS_CMD."Close" ("State")) -> ("error out"=w272:errorcluster)  [unwired: 12 in, 5 out]
            n197 = call "(Instrl) HVPS_1.vi"("IP"=w276, "Port"=w275, "error in (no error)"=w272, "CMD"=(Ctrl)_State_HVPS_CMD."Open" ("State")) -> ("error out"=w277:errorcluster)  [unwired: 10 in, 5 out]
          }
        }
        n198 = case shown="에러" w255 {
          selector: w255 -> [w279 w281]
          tunnel: [w279 w281] -> w258
          frame No Error {
          }
          frame Error {
            n199 = global read "(Var) Get_HVPS_1.vi" "G1. Stop"() -> (w280:bool)
            n200 = local write "G1_TEST END?"(w280) -> ()
          }
        }
        n201 = Select(t=(Ctrl)_State_Test_Manage."Run Init" ("State"), s=w261, f=(Ctrl)_State_Test_Manage."Idls" ("State")) -> (s? t:f=w260:T1)
        n202 = Select(t=(Ctrl)_State_Test_Manage."Idls" ("State"), s=w258, f=w260) -> (s? t:f=w257:T1)
        n203 = local read "Exit ?"() -> (w266:bool)
        n204 = Select(t=(Ctrl)_State_Test_Manage."Close" ("State"), s=w266, f=w257) -> (s? t:f=w263:T1)
      }
      frame "Run Init" {
        n205 = flat-sequence {
          tunnel: w305 -> [w324]
          tunnel: [w324] -> w304
          tunnel: [w332] -> w303
          tunnel: w304 -> [w332]
          frame #0 {
            w321 = 0.0 ("G1. KV")
            n206 = global write "(Var) Get_HVPS_1.vi" "G1. mA"(w321) -> ()
            n207 = global write "(Var) Get_HVPS_1.vi" "G1. KV"(w321) -> ()
            n208 = call "(Sub) Falling Step.vi"("State"=T9."G1. Reset") -> ()  [unwired: 7 in, 4 out]
            n209 = property on="G1. Voltage Graph" class="WFChart (엄격한)"("History Data"=dbl[] [] ("히스토리 데이터")) -> ()  [unwired: 2 in, 2 out]
            n210 = property on="G1. Current Graph" class="WFChart (엄격한)"("History Data"=T10 [] ("히스토리 데이터")) -> ()  [unwired: 2 in, 2 out]
          }
          frame #1 {
            n211 = property on="G1. Start Butten" class="Bool"("DisabledEnum"=T7."Disabled and Grayed Out" ("비활성화")) -> ()  [unwired: 2 in, 2 out]
            n212 = property on="G1. Stop Butten" class="Bool"("DisabledEnum"=T7."Enabled" ("비활성화")) -> ()  [unwired: 2 in, 2 out]
            n213 = property on="G1. Taget Voltage" class="DigNum (엄격한)"("DisabledEnum"=T7."Disabled and Grayed Out" ("비활성화")) -> ()  [unwired: 2 in, 2 out]
            n214 = property on="Group1. Info" class="Str"("DisabledEnum"=T7."Disabled and Grayed Out" ("비활성화")) -> ()  [unwired: 2 in, 2 out]
            n215 = property on="G1. Current Limit" class="DigNum (엄격한)"("DisabledEnum"=T7."Disabled and Grayed Out" ("비활성화")) -> ()  [unwired: 2 in, 2 out]
            n216 = property on="G1. Start Delay" class="DigNum (엄격한)"("DisabledEnum"=T7."Disabled and Grayed Out" ("비활성화")) -> ()  [unwired: 2 in, 2 out]
            n217 = property on="G1. Delay" class="DigNum (엄격한)"("Visible"=TRUE ("보이기")) -> ()  [unwired: 2 in, 2 out]
          }
        }
        n218 = local write "G1. Test  Status"(u16 7 ("G1. Test  Status")) -> ()
        n219 = Get Date/Time In Seconds() -> (seconds since 1Jan1904=w302:timestamp)
        n220 = while {
          tunnel: w303 -> [w319]
          tunnel: [w319] -> w297
          tunnel: w302 -> [w318]
          stop <- w314 stop-if-true
          n221 = local read "G1. Start Delay"() -> (w313:dbl)
          n222 = Get Date/Time In Seconds() -> (seconds since 1Jan1904=w317:timestamp)
          n223 = Subtract(x=w317, y=w318) -> (x-y=w312:dbl)
          n224 = global read "(Var) Get_HVPS_1.vi" "G1. Stop"() -> (w310:bool)
          n225 = Greater Or Equal?(x=w312, y=w313) -> (x >= y?=w316:bool)
          n226 = Subtract(x=w313, y=w312) -> (x-y=→"G1. Delay":dbl)
          n227 = Or(x=w316, y=w310) -> (x .or. y?=w314:bool)
          n228 = Wait (ms)(milliseconds to wait=u32 1 ("대기 시간 (ms)")) -> ()  [unwired: 1 out]
        }
        n229 = flat-sequence {
          tunnel: [w309] -> w300
          tunnel: w297 -> [_]
          frame #0 {
            n230 = global read "(Var) Get_HVPS_1.vi" "G1. Stop"() -> (w306:bool)
            n231 = Select(t=(Ctrl)_State_Test_Manage."Falling" ("State"), s=w306, f=(Ctrl)_State_Test_Manage."Rising" ("State")) -> (s? t:f=w309:T1)
          }
        }
        n232 = property on="G1. Delay" class="DigNum (엄격한)"(error in=w297, "Visible"=FALSE ("보이기")) -> (error out=w298:errorcluster)  [unwired: 1 in, 1 out]
      }
      frame "Run" {
        # "Limit 값 넘으면, Quick Stop\nQuick Stop 버튼 누르면, Quick Stop\nExit 버튼 누르면, Quick Stop\nStop 버튼 누르면, Stop"
        n233 = local read "G1.Comm"() -> (w350:bool)
        n234 = local write "G1. Test  Status"(u16 2 ("G1. Test  Status")) -> ()
        n235 = call "경과 시간3"("Reset"=w342, "Auto Reset"=FALSE) -> ("Elapsed Time (s)"=w340:dbl)  [unwired: 10 in, 7 out]
        n236 = local read "G1. Current Limit"() -> (w344:dbl)
        n237 = local read "G1. Target Time"() -> (w341:dbl)
        n238 = global read "(Var) Get_HVPS_1.vi" "G1. mA"() -> (w333:dbl)
        n239 = local write "G1. Time"(w340) -> ()
        n240 = Greater Or Equal?(x=w333, y=w344) -> (x >= y?=w356:bool)
        n241 = Greater Or Equal?(x=w340, y=w341) -> (x >= y?=w338:bool)
        n242 = Wait Until Next ms Multiple(millisecond multiple=u32 300 ("대기 시간 (ms)")) -> ()  [unwired: 1 out]
        n243 = Select(t=(Ctrl)_State_Test_Manage."Idls" ("State"), s=w350, f=(Ctrl)_State_Test_Manage."Run" ("State")) -> (s? t:f=w348:T1)
        n244 = Select(t=(Ctrl)_State_Test_Manage."Quick Falling" ("State"), s=w356, f=w348) -> (s? t:f=w354:T1)
        n245 = global read "(Var) Get_HVPS_1.vi" "G1. Start"() -> (w335:bool)
        n246 = Select(t=w354, s=w335, f=(Ctrl)_State_Test_Manage."Falling" ("State")) -> (s? t:f=w339:T1)
        n247 = global read "(Var) Get_HVPS_1.vi" "G1. Q Stop"() -> (w334:bool)
        n248 = Select(t=(Ctrl)_State_Test_Manage."Falling" ("State"), s=w338, f=w339) -> (s? t:f=w336:T1)
        n249 = Select(t=(Ctrl)_State_Test_Manage."Quick Falling" ("State"), s=w334, f=w336) -> (s? t:f=w346:T1)
      }
      frame "Rising" {
        n250 = stacked-sequence {
          tunnel: w369 -> [_ _ _ _]
          tunnel: [w392 _ _ _] -> w367
          tunnel: [_ w398 _ _] -> w366
          tunnel: [_ _ w403 _] -> w365
          tunnel: [_ _ _ w409] -> w364
          frame #0 {
            w395 = 0.0  # Set V
            # "0V SET"
            n251 = call "(Sub) CMD Parsing_1.vi"("Set V"=w395, "State"=(Ctrl)_State_Parcing."Set V") -> ("CMD Set V"=w391:string, "error out"=w396:errorcluster)  [unwired: 9 in, 3 out]
            n252 = call "(Instrl) HVPS_1.vi"("Write Data"=w391, "error in (no error)"=w396, "CMD"=(Ctrl)_State_HVPS_CMD."Tx : Set V" ("State")) -> ("error out"=w392:errorcluster)  [unwired: 11 in, 5 out]
          }
          frame #1 {
            w400 = 0.0  # Set mA
            # "0mA SET"
            n253 = call "(Sub) CMD Parsing_1.vi"("State"=(Ctrl)_State_Parcing."Set mA", "Set mA"=w400) -> ("CMD Set mA"=w399:string, "error out"=w402:errorcluster)  [unwired: 9 in, 3 out]
            n254 = call "(Instrl) HVPS_1.vi"("Write Data"=w399, "error in (no error)"=w402, "CMD"=(Ctrl)_State_HVPS_CMD."Tx : Set mA" ("State")) -> ("error out"=w398:errorcluster)  [unwired: 11 in, 5 out]
          }
          frame #2 {
            # "Power ON"
            n255 = call "(Instrl) HVPS_1.vi"("CMD"=(Ctrl)_State_HVPS_CMD."Tx : ON" ("State")) -> ("error out"=w403:errorcluster)  [unwired: 13 in, 5 out]
          }
          frame #3 {
            # "mA SET"
            n256 = local read "G1. Current Limit"() -> (w406:dbl)
            n257 = call "(Sub) CMD Parsing_1.vi"("State"=(Ctrl)_State_Parcing."Set mA", "Set mA"=w406) -> ("CMD Set mA"=w407:string, "error out"=w411:errorcluster)  [unwired: 9 in, 3 out]
            n258 = call "(Instrl) HVPS_1.vi"("Write Data"=w407, "error in (no error)"=w411, "CMD"=(Ctrl)_State_HVPS_CMD."Tx : Set mA" ("State")) -> ("error out"=w409:errorcluster)  [unwired: 11 in, 5 out]
            n259 = Wait (ms)(milliseconds to wait=u32 300 ("대기 시간 (ms)")) -> ()  [unwired: 1 out]
          }
        }
        n260 = local write "G1. Test  Status"(u16 3 ("G1. Test  Status")) -> ()
        n261 = local read "G1. Taget Voltage"() -> (w360:dbl)
        n262 = Merge Errors(w367, w366, w365, w364) -> (w363:errorcluster)
        n263 = call "(Sub) Power Sweep.vi"("Taget Voltage"=w360) -> ("ON Sweep"=w361:dbl[])  [unwired: 8 in, 2 out]
        n264 = case shown="에러 없음" w363 {
          selector: w363 -> [w372 _]
          tunnel: w361 -> [w371 w390]
          tunnel: [w370 w390] -> w357
          frame No Error {
            n265 = for {
              tunnel: w372 -> [w381]
              tunnel: w371 -> [w373] mode=indexing
              tunnel: [w373] -> w370 mode=indexing
              stop <- w377 stop-if-true
              n266 = call "(Sub) CMD Parsing_1.vi"("Set V"=w373, "State"=(Ctrl)_State_Parcing."Set V", "error in (no error)"=w381) -> ("CMD Set V"=w376:string, "error out"=w380:errorcluster)  [unwired: 8 in, 3 out]
              n267 = call "(Instrl) HVPS_1.vi"("Write Data"=w376, "error in (no error)"=w380, "CMD"=(Ctrl)_State_HVPS_CMD."Tx : Set V") -> ("error out"=w378:errorcluster)  [unwired: 11 in, 5 out]
              n268 = while {
                shift-right: [FALSE] -> _
                shift-left: TRUE -> [w388]
                tunnel: w378 -> [_]
                tunnel: [w382] -> w377
                stop <- w384 stop-if-true
                n269 = global read "(Var) Get_HVPS_1.vi" "G1. Stop"() -> (w382:bool)
                n270 = call "경과 시간"("Time Target (s)"=5.0, "Reset"=w388, "Auto Reset"=FALSE) -> ("Time has Elapsed"=w386:bool)  [unwired: 9 in, 7 out]
                n271 = Wait Until Next ms Multiple(millisecond multiple=u32 1 ("ms 배수")) -> ()  [unwired: 1 out]
                n272 = Compound Arithmetic op=OR ("복합 연산")(w386, w382) -> (w384:bool)
              }
            }
          }
          frame Error {
          }
        }
        n273 = call "(Sub) Falling Step.vi"("State"=T9."G1. Save", "G1. Rising Step"=w357) -> ()  [unwired: 6 in, 4 out]
      }
      frame "Falling" {
        n274 = local write "G1. Test  Status"(u16 4 ("G1. Test  Status")) -> ()
        n275 = call "(Sub) Falling Step.vi"("State"=T9."G1. Load") -> ("G1. Falling Step"=w412:dbl[])  [unwired: 7 in, 3 out]
        n276 = Reverse 1D Array(array=w412) -> (reversed array=w420:dbl[])
        n277 = Build Array (concatenate)(w420, 0.0) -> (w417:dbl[])
        n278 = Delete From Array(array=w417, length=1 ("길이"), index=0 ("인덱스")) -> (array with subset deleted=w416:dbl[])  [unwired: 1 out]
        n279 = for {
          tunnel: w425 -> [w437]
          tunnel: w416 -> [w438] mode=indexing
          tunnel: [errorcluster {"status"=FALSE, "code"=0, "source"=""} ("에러 상수")] -> w424
          stop <- w433 stop-if-true
          n280 = call "(Sub) CMD Parsing_1.vi"("Set V"=w438, "State"=(Ctrl)_State_Parcing."Set V", "error in (no error)"=w437) -> ("CMD Set V"=w430:string, "error out"=w436:errorcluster)  [unwired: 8 in, 3 out]
          n281 = call "(Instrl) HVPS_1.vi"("Write Data"=w430, "error in (no error)"=w436, "CMD"=(Ctrl)_State_HVPS_CMD."Tx : Set V" ("State")) -> ("error out"=w434:errorcluster)  [unwired: 11 in, 5 out]
          n282 = while {
            shift-right: [FALSE] -> _
            shift-left: TRUE -> [w448]
            tunnel: w434 -> [_]
            tunnel: [w443] -> w433
            stop <- w444 stop-if-true
            n283 = global read "(Var) Get_HVPS_1.vi" "G1. Q Stop"() -> (w440:bool)
            n284 = local read "G1.Comm"() -> (w442:bool)
            n285 = call "경과 시간2"("Time Target (s)"=5.0, "Reset"=w448, "Auto Reset"=FALSE) -> ("Time has Elapsed"=w446:bool)  [unwired: 9 in, 7 out]
            n286 = Wait Until Next ms Multiple(millisecond multiple=u32 1 ("ms 배수")) -> ()  [unwired: 1 out]
            n287 = Compound Arithmetic op=OR ("복합 연산")(w442, w446, w440) -> (w444:bool)
            n288 = Compound Arithmetic op=OR ("복합 연산")(w442, w440) -> (w443:bool)
          }
        }
        n289 = global read "(Var) Get_HVPS_1.vi" "G1. Q Stop"() -> (w414:bool)
        n290 = case shown="거짓" w414 {
          tunnel: w424 -> [w453 _]
          tunnel: [w450 errorcluster {"status"=FALSE, "code"=0, "source"=""} ("에러 상수")] -> w415
          frame False {
            n291 = stacked-sequence {
              tunnel: w453 -> [_ _ _ _]
              tunnel: [w455 _ _ _] -> w451
              tunnel: [_ w460 _ _] -> w452
              frame #0 {
                w457 = 0.0  # Set mA
                # "0mA SET"
                n292 = call "(Sub) CMD Parsing_1.vi"("State"=(Ctrl)_State_Parcing."Set mA", "Set mA"=w457) -> ("CMD Set mA"=w456:string, "error out"=w459:errorcluster)  [unwired: 9 in, 3 out]
                n293 = call "(Instrl) HVPS_1.vi"("Write Data"=w456, "error in (no error)"=w459, "CMD"=(Ctrl)_State_HVPS_CMD."Tx : Set mA" ("State")) -> ("error out"=w455:errorcluster)  [unwired: 11 in, 5 out]
              }
              frame #1 {
                # "Power OFF"
                n294 = call "(Instrl) HVPS_1.vi"("CMD"=(Ctrl)_State_HVPS_CMD."Tx : OFF" ("State")) -> ("error out"=w460:errorcluster)  [unwired: 13 in, 5 out]
              }
              frame #2 {
                n295 = local write "G1_TEST END?"(TRUE ("G1_TEST END?")) -> ()
                n296 = local write "G1. Test  Status"(u16 5 ("Test END")) -> ()
                n297 = global write "(Var) Get_HVPS_1.vi" "G1. Stop"(TRUE ("G1. Stop")) -> ()
                n298 = global write "(Var) Get_HVPS_1.vi" "G1. Start"(FALSE ("G1. Start")) -> ()
              }
              frame #3 {
                n299 = property on="Group1. Info" class="Str"("DisabledEnum"=T7."Enabled" ("비활성화")) -> ()  [unwired: 2 in, 2 out]
                n300 = property on="G1. Start Delay" class="DigNum (엄격한)"("DisabledEnum"=T7."Enabled" ("비활성화")) -> ()  [unwired: 2 in, 2 out]
                n301 = property on="G1. Start Butten" class="Bool"("DisabledEnum"=T7."Enabled" ("비활성화")) -> ()  [unwired: 2 in, 2 out]
                n302 = property on="G1. Stop Butten" class="Bool"("DisabledEnum"=T7."Disabled and Grayed Out" ("비활성화")) -> ()  [unwired: 2 in, 2 out]
                n303 = property on="G1. Taget Voltage" class="DigNum (엄격한)"("DisabledEnum"=T7."Enabled" ("비활성화")) -> ()  [unwired: 2 in, 2 out]
                n304 = property on="G1. Current Limit" class="DigNum (엄격한)"("DisabledEnum"=T7."Enabled" ("비활성화")) -> ()  [unwired: 2 in, 2 out]
              }
            }
            n305 = Merge Errors(w451, w452) -> (w450:errorcluster)
          }
          frame True {
          }
        }
        n306 = flat-sequence {
          tunnel: [w429] -> w423
          tunnel: w415 -> [_]
          frame #0 {
            n307 = global read "(Var) Get_HVPS_1.vi" "G1. Q Stop"() -> (w426:bool)
            n308 = Select(t=(Ctrl)_State_Test_Manage."Quick Falling" ("State"), s=w426, f=(Ctrl)_State_Test_Manage."Idls" ("State")) -> (s? t:f=w429:T1)
          }
        }
      }
      frame "Quick Falling" {
        n309 = local write "G1. Test  Status"(u16 6 ("G1. Test  Status")) -> ()
        n310 = stacked-sequence {
          tunnel: [_ _ w495 _ _] -> w475
          tunnel: w482 -> [_ _ _ _ _]
          tunnel: [w484 _ _ _ _] -> w477
          tunnel: [_ w490 _ _ _] -> w476
          frame #0 {
            w486 = 0.0  # Set V
            # "0V SET"
            n311 = call "(Sub) CMD Parsing_1.vi"("Set V"=w486, "State"=(Ctrl)_State_Parcing."Set V") -> ("CMD Set V"=w485:string, "error out"=w488:errorcluster)  [unwired: 9 in, 3 out]
            n312 = call "(Instrl) HVPS_1.vi"("Write Data"=w485, "error in (no error)"=w488, "CMD"=(Ctrl)_State_HVPS_CMD."Tx : Set V" ("State")) -> ("error out"=w484:errorcluster)  [unwired: 11 in, 5 out]
          }
          frame #1 {
            w492 = 0.0  # Set mA
            # "0mA SET"
            n313 = call "(Sub) CMD Parsing_1.vi"("State"=(Ctrl)_State_Parcing."Set mA", "Set mA"=w492) -> ("CMD Set mA"=w491:string, "error out"=w494:errorcluster)  [unwired: 9 in, 3 out]
            n314 = call "(Instrl) HVPS_1.vi"("Write Data"=w491, "error in (no error)"=w494, "CMD"=(Ctrl)_State_HVPS_CMD."Tx : Set mA" ("State")) -> ("error out"=w490:errorcluster)  [unwired: 11 in, 5 out]
          }
          frame #2 {
            # "Power OFF"
            n315 = call "(Instrl) HVPS_1.vi"("CMD"=(Ctrl)_State_HVPS_CMD."Tx : OFF" ("State")) -> ("error out"=w495:errorcluster)  [unwired: 13 in, 5 out]
          }
          frame #3 {
            w500 = u16 6  # Shutdown
            n316 = local write "G1. Test  Status"(w500) -> ()
            n317 = global write "(Var) Get_HVPS_1.vi" "G1. Start"(FALSE ("G1. Start")) -> ()
            n318 = local write "G1_TEST END?"(TRUE ("G1_TEST END?")) -> ()
            n319 = global write "(Var) Get_HVPS_1.vi" "G1. Stop"(TRUE ("G1. Stop")) -> ()
          }
          frame #4 {
            n320 = property on="G1. Start Butten" class="Bool"("DisabledEnum"=T7."Enabled" ("비활성화")) -> ()  [unwired: 2 in, 2 out]
            n321 = property on="G1. Stop Butten" class="Bool"("DisabledEnum"=T7."Disabled and Grayed Out" ("비활성화")) -> ()  [unwired: 2 in, 2 out]
            n322 = property on="G1. Taget Voltage" class="DigNum (엄격한)"("DisabledEnum"=T7."Enabled" ("비활성화")) -> ()  [unwired: 2 in, 2 out]
            n323 = property on="G1. Current Limit" class="DigNum (엄격한)"("DisabledEnum"=T7."Enabled" ("비활성화")) -> ()  [unwired: 2 in, 2 out]
            n324 = property on="Group1. Info" class="Str"("DisabledEnum"=T7."Enabled" ("비활성화")) -> ()  [unwired: 2 in, 2 out]
            n325 = property on="G1. Start Delay" class="DigNum (엄격한)"("DisabledEnum"=T7."Enabled" ("비활성화")) -> ()  [unwired: 2 in, 2 out]
          }
        }
        n326 = Merge Errors(w477, w476, w475) -> (w474:errorcluster)
        n327 = local read "Exit ?"() -> (w481:bool)
        n328 = Select(t=(Ctrl)_State_Test_Manage."Close" ("State"), s=w481, f=(Ctrl)_State_Test_Manage."Idls" ("State")) -> (s? t:f=w480:T1)
      }
      frame "Close" {
        n329 = flat-sequence {
          tunnel: [w511] -> w508
          tunnel: w507 -> [_]
          frame #0 {
            n330 = call "(Instrl) HVPS_1.vi"("CMD"=(Ctrl)_State_HVPS_CMD."Close" ("State")) -> ("error out"=w511:errorcluster)  [unwired: 13 in, 5 out]
          }
        }
      }
    }
    "G1. State" <- w253
  }
  n331 = while "Group.2 HVPS Manager Loop" {
    shift-right: [w519] -> _
    shift-left: (Ctrl)_State_Test_Manage."Idls" ("State") -> [w515]
    tunnel: w1 -> [w516]
    tunnel: [w517] -> w6
    shift-right: [w513] -> _
    shift-left: _ -> [w514]
    stop <- w518 stop-if-true
    n332 = case shown="\"Run\"" w515 {
      tunnel: [w529 w567 w612 (Ctrl)_State_Test_Manage."Run" ("State") w688 w745 (Ctrl)_State_Test_Manage."Close" ("State")] -> w519
      tunnel: [_ _ _ _ _ _ TRUE] -> w518
      tunnel: w516 -> [w533 w571 _ w635 w690 w747 w772]
      tunnel: [_ w564 _ _ w680 w739 w773] -> w517
      tunnel: w514 -> [_ _ w606 _ _ _ _]
      tunnel: [_ _ _ TRUE _ _ _] -> w513
      frame "Idls", Default {
        n333 = flat-sequence {
          tunnel: w533 -> [w556]
          tunnel: [w555] -> w535
          tunnel: [w556] -> w534
          tunnel: [w562] -> w528
          tunnel: w535 -> [w559]
          tunnel: w534 -> [w562]
          tunnel: [w557] -> w527
          frame #0 {
            n334 = global read "(Var) Get_HVPS_2.vi" "G2. Start"() -> (w555:bool)
          }
          frame #1 {
            n335 = local read "G2_TEST END?"() -> (w560:bool)
            n336 = Wait (ms)(milliseconds to wait=u32 300 ("대기 시간 (ms)")) -> ()  [unwired: 1 out]
            n337 = Select(t=FALSE, s=w560, f=w559) -> (s? t:f=w557:bool)
          }
        }
        n338 = local read "G2_TEST END?"() -> (w522:bool)
        n339 = case shown="거짓" w522 {
          frame False {
            w549 = 1  # Ready
            w550 = 0  # NOT Ready
            n340 = local read "G2.System"() -> (w553:bool)
            n341 = local read "G2.Comm"() -> (w554:bool)
            n342 = Compound Arithmetic op=AND(w554, w553, TRUE) -> (w551:bool)
            n343 = Select(t=w550, s=w551, f=w549) -> (s? t:f=w548:i32)
            n344 = local write "G2. Test  Status"(w548) -> ()
          }
          frame True {
          }
        }
        n345 = local read "G2.Comm"() -> (w520:bool)
        n346 = case shown="거짓" w520 {
          tunnel: w528 -> [w537 w540]
          tunnel: [w537 w543] -> w521
          frame False {
          }
          frame True {
            w541 = u16 50001  # Port
            w542 = "192.168.10.62"  # IP
            n347 = call "(Instrl) HVPS_2.vi"("error in (no error)"=w540, "CMD"=(Ctrl)_State_HVPS_CMD."Close" ("State")) -> ("error out"=w538:errorcluster)  [unwired: 12 in, 5 out]
            n348 = call "(Instrl) HVPS_2.vi"("IP"=w542, "Port"=w541, "error in (no error)"=w538, "CMD"=(Ctrl)_State_HVPS_CMD."Open" ("State")) -> ("error out"=w543:errorcluster)  [unwired: 10 in, 5 out]
          }
        }
        n349 = case shown="에러" w521 {
          selector: w521 -> [w545 w547]
          tunnel: [w545 w547] -> w524
          frame No Error {
          }
          frame Error {
            n350 = global read "(Var) Get_HVPS_2.vi" "G2. Stop"() -> (w546:bool)
            n351 = local write "G2_TEST END?"(w546) -> ()
          }
        }
        n352 = Select(t=(Ctrl)_State_Test_Manage."Run Init" ("State"), s=w527, f=(Ctrl)_State_Test_Manage."Idls" ("State")) -> (s? t:f=w526:T1)
        n353 = Select(t=(Ctrl)_State_Test_Manage."Idls" ("State"), s=w524, f=w526) -> (s? t:f=w523:T1)
        n354 = local read "Exit ?"() -> (w532:bool)
        n355 = Select(t=(Ctrl)_State_Test_Manage."Close" ("State"), s=w532, f=w523) -> (s? t:f=w529:T1)
      }
      frame "Run Init" {
        n356 = flat-sequence {
          tunnel: w571 -> [w590]
          tunnel: [w590] -> w570
          tunnel: [w598] -> w568
          tunnel: w570 -> [w598]
          frame #0 {
            w587 = 0.0 ("G1. KV")
            n357 = global write "(Var) Get_HVPS_2.vi" "G2. mA"(w587) -> ()
            n358 = global write "(Var) Get_HVPS_2.vi" "G2. KV"(w587) -> ()
            n359 = call "(Sub) Falling Step.vi"("State"=T9."G2. Reset") -> ()  [unwired: 7 in, 4 out]
            n360 = property on="G2. Voltage Graph" class="WFChart (엄격한)"("History Data"=dbl[] [] ("히스토리 데이터")) -> ()  [unwired: 2 in, 2 out]
            n361 = property on="G2. Current Graph" class="WFChart (엄격한)"("History Data"=T10 [] ("히스토리 데이터")) -> ()  [unwired: 2 in, 2 out]
          }
          frame #1 {
            n362 = property on="G2. Delay" class="DigNum (엄격한)"("Visible"=TRUE ("보이기")) -> ()  [unwired: 2 in, 2 out]
            n363 = property on="G2. Start Delay" class="DigNum (엄격한)"("DisabledEnum"=T7."Disabled and Grayed Out" ("비활성화")) -> ()  [unwired: 2 in, 2 out]
            n364 = property on="Group2. Info" class="Str"("DisabledEnum"=T7."Disabled and Grayed Out" ("비활성화")) -> ()  [unwired: 2 in, 2 out]
            n365 = property on="G2. Start Butten" class="Bool"("DisabledEnum"=T7."Disabled and Grayed Out" ("비활성화")) -> ()  [unwired: 2 in, 2 out]
            n366 = property on="G2. Stop Butten" class="Bool"("DisabledEnum"=T7."Enabled" ("비활성화")) -> ()  [unwired: 2 in, 2 out]
            n367 = property on="G2. Taget Voltage" class="DigNum (엄격한)"("DisabledEnum"=T7."Disabled and Grayed Out" ("비활성화")) -> ()  [unwired: 2 in, 2 out]
            n368 = property on="G2. Current Limit" class="DigNum (엄격한)"("DisabledEnum"=T7."Disabled and Grayed Out" ("비활성화")) -> ()  [unwired: 2 in, 2 out]
          }
        }
        n369 = local write "G2. Test  Status"(u16 7 ("G1. Test  Status")) -> ()
        n370 = Get Date/Time In Seconds() -> (seconds since 1Jan1904=w569:timestamp)
        n371 = while {
          tunnel: w568 -> [w585]
          tunnel: [w585] -> w563
          tunnel: w569 -> [w584]
          stop <- w580 stop-if-true
          n372 = local read "G2. Start Delay"() -> (w579:dbl)
          n373 = Get Date/Time In Seconds() -> (seconds since 1Jan1904=w583:timestamp)
          n374 = Subtract(x=w583, y=w584) -> (x-y=w578:dbl)
          n375 = global read "(Var) Get_HVPS_2.vi" "G2. Stop"() -> (w576:bool)
          n376 = Greater Or Equal?(x=w578, y=w579) -> (x >= y?=w582:bool)
          n377 = Subtract(x=w579, y=w578) -> (x-y=→"G2. Delay":dbl)
          n378 = Or(x=w582, y=w576) -> (x .or. y?=w580:bool)
          n379 = Wait (ms)(milliseconds to wait=u32 1 ("대기 시간 (ms)")) -> ()  [unwired: 1 out]
        }
        n380 = flat-sequence {
          tunnel: [w573] -> w567
          tunnel: w563 -> [_]
          frame #0 {
            n381 = global read "(Var) Get_HVPS_2.vi" "G2. Stop"() -> (w572:bool)
            n382 = Select(t=(Ctrl)_State_Test_Manage."Falling" ("State"), s=w572, f=(Ctrl)_State_Test_Manage."Rising" ("State")) -> (s? t:f=w573:T1)
          }
        }
        n383 = property on="G2. Delay" class="DigNum (엄격한)"(error in=w563, "Visible"=FALSE ("보이기")) -> (error out=w564:errorcluster)  [unwired: 1 in, 1 out]
      }
      frame "Run" {
        # "Limit 값 넘으면, Quick Stop\nQuick Stop 버튼 누르면, Quick Stop\nExit 버튼 누르면, Quick Stop\nStop 버튼 누르면, Stop"
        n384 = local read "G2.Comm"() -> (w616:bool)
        n385 = local write "G2. Test  Status"(u16 2 ("G1. Test  Status")) -> ()
        n386 = local read "G2. Current Limit"() -> (w610:dbl)
        n387 = call "경과 시간9"("Reset"=w606, "Auto Reset"=FALSE) -> ("Elapsed Time (s)"=w609:dbl)  [unwired: 10 in, 7 out]
        n388 = global read "(Var) Get_HVPS_2.vi" "G2. mA"() -> (w599:dbl)
        n389 = local read "G2. Target Time"() -> (w608:dbl)
        n390 = local write "G2. Time"(w609) -> ()
        n391 = Greater Or Equal?(x=w599, y=w610) -> (x >= y?=w622:bool)
        n392 = Wait Until Next ms Multiple(millisecond multiple=u32 300 ("대기 시간 (ms)")) -> ()  [unwired: 1 out]
        n393 = Greater Or Equal?(x=w609, y=w608) -> (x >= y?=w603:bool)
        n394 = Select(t=(Ctrl)_State_Test_Manage."Idls" ("State"), s=w616, f=(Ctrl)_State_Test_Manage."Run" ("State")) -> (s? t:f=w614:T1)
        n395 = Select(t=(Ctrl)_State_Test_Manage."Quick Falling" ("State"), s=w622, f=w614) -> (s? t:f=w620:T1)
        n396 = global read "(Var) Get_HVPS_2.vi" "G2. Start"() -> (w601:bool)
        n397 = Select(t=w620, s=w601, f=(Ctrl)_State_Test_Manage."Falling" ("State")) -> (s? t:f=w605:T1)
        n398 = global read "(Var) Get_HVPS_2.vi" "G2. Q Stop"() -> (w600:bool)
        n399 = Select(t=(Ctrl)_State_Test_Manage."Falling" ("State"), s=w603, f=w605) -> (s? t:f=w604:T1)
        n400 = Select(t=(Ctrl)_State_Test_Manage."Quick Falling" ("State"), s=w600, f=w604) -> (s? t:f=w612:T1)
      }
      frame "Rising" {
        n401 = stacked-sequence {
          tunnel: w635 -> [_ _ _ _]
          tunnel: [w658 _ _ _] -> w633
          tunnel: [_ w664 _ _] -> w632
          tunnel: [_ _ w669 _] -> w631
          tunnel: [_ _ _ w674] -> w630
          frame #0 {
            w661 = 0.0  # Set V
            # "0V SET"
            n402 = call "(Sub) CMD Parsing_2.vi"("Set V"=w661, "State"=(Ctrl)_State_Parcing."Set V") -> ("CMD Set V"=w657:string, "error out"=w662:errorcluster)  [unwired: 9 in, 3 out]
            n403 = call "(Instrl) HVPS_2.vi"("Write Data"=w657, "error in (no error)"=w662, "CMD"=(Ctrl)_State_HVPS_CMD."Tx : Set V" ("State")) -> ("error out"=w658:errorcluster)  [unwired: 11 in, 5 out]
          }
          frame #1 {
            w666 = 0.0  # Set mA
            # "0mA SET"
            n404 = call "(Sub) CMD Parsing_2.vi"("State"=(Ctrl)_State_Parcing."Set mA", "Set mA"=w666) -> ("CMD Set mA"=w665:string, "error out"=w668:errorcluster)  [unwired: 9 in, 3 out]
            n405 = call "(Instrl) HVPS_2.vi"("Write Data"=w665, "error in (no error)"=w668, "CMD"=(Ctrl)_State_HVPS_CMD."Tx : Set mA" ("State")) -> ("error out"=w664:errorcluster)  [unwired: 11 in, 5 out]
          }
          frame #2 {
            # "Power ON"
            n406 = call "(Instrl) HVPS_2.vi"("CMD"=(Ctrl)_State_HVPS_CMD."Tx : ON" ("State")) -> ("error out"=w669:errorcluster)  [unwired: 13 in, 5 out]
          }
          frame #3 {
            # "mA SET"
            n407 = local read "G2. Current Limit"() -> (w671:dbl)
            n408 = call "(Sub) CMD Parsing_2.vi"("State"=(Ctrl)_State_Parcing."Set mA", "Set mA"=w671) -> ("CMD Set mA"=w672:string, "error out"=w676:errorcluster)  [unwired: 9 in, 3 out]
            n409 = call "(Instrl) HVPS_2.vi"("Write Data"=w672, "error in (no error)"=w676, "CMD"=(Ctrl)_State_HVPS_CMD."Tx : Set mA" ("State")) -> ("error out"=w674:errorcluster)  [unwired: 11 in, 5 out]
          }
        }
        n410 = local write "G2. Test  Status"(u16 3 ("G1. Test  Status")) -> ()
        n411 = local read "G2. Taget Voltage"() -> (w627:dbl)
        n412 = Merge Errors(w633, w632, w631, w630) -> (w629:errorcluster)
        n413 = call "(Sub) Power Sweep.vi"("Taget Voltage"=w627) -> ("ON Sweep"=w626:dbl[])  [unwired: 8 in, 2 out]
        n414 = case shown="에러 없음" w629 {
          selector: w629 -> [w637 _]
          tunnel: w626 -> [w638 w656]
          tunnel: [w636 w656] -> w623
          frame No Error {
            n415 = for {
              tunnel: w637 -> [w646]
              tunnel: w638 -> [w639] mode=indexing
              tunnel: [w639] -> w636 mode=indexing
              stop <- w642 stop-if-true
              n416 = call "(Sub) CMD Parsing_2.vi"("Set V"=w639, "State"=(Ctrl)_State_Parcing."Set V", "error in (no error)"=w646) -> ("CMD Set V"=w640:string, "error out"=w645:errorcluster)  [unwired: 8 in, 3 out]
              n417 = call "(Instrl) HVPS_2.vi"("Write Data"=w640, "error in (no error)"=w645, "CMD"=(Ctrl)_State_HVPS_CMD."Tx : Set V" ("State")) -> ("error out"=w643:errorcluster)  [unwired: 11 in, 5 out]
              n418 = while {
                shift-right: [FALSE] -> _
                shift-left: TRUE -> [w654]
                tunnel: w643 -> [_]
                tunnel: [w648] -> w642
                stop <- w650 stop-if-true
                n419 = global read "(Var) Get_HVPS_2.vi" "G2. Stop"() -> (w648:bool)
                n420 = call "경과 시간4"("Time Target (s)"=5.0, "Reset"=w654, "Auto Reset"=FALSE) -> ("Time has Elapsed"=w652:bool)  [unwired: 9 in, 7 out]
                n421 = Wait Until Next ms Multiple(millisecond multiple=u32 1 ("ms 배수")) -> ()  [unwired: 1 out]
                n422 = Or(x=w652, y=w648) -> (x .or. y?=w650:bool)
              }
            }
          }
          frame Error {
          }
        }
        n423 = call "(Sub) Falling Step.vi"("State"=T9."G2. Save", "G2. Rising Step"=w623) -> ()  [unwired: 6 in, 4 out]
      }
      frame "Falling" {
        n424 = local write "G2. Test  Status"(u16 4 ("G1. Test  Status")) -> ()
        n425 = call "(Sub) Falling Step.vi"("State"=T9."G2. Load") -> ("G2. Falling Step"=w677:dbl[])  [unwired: 7 in, 3 out]
        n426 = Reverse 1D Array(array=w677) -> (reversed array=w685:dbl[])
        n427 = Build Array (concatenate)(w685, 0.0) -> (w682:dbl[])
        n428 = Delete From Array(array=w682, length=1 ("길이"), index=0 ("인덱스")) -> (array with subset deleted=w681:dbl[])  [unwired: 1 out]
        n429 = for {
          tunnel: w690 -> [w725]
          tunnel: w681 -> [w726] mode=indexing
          tunnel: [errorcluster {"status"=FALSE, "code"=0, "source"=""} ("에러 상수")] -> w689
          stop <- w721 stop-if-true
          n430 = call "(Sub) CMD Parsing_2.vi"("Set V"=w726, "State"=(Ctrl)_State_Parcing."Set V", "error in (no error)"=w725) -> ("CMD Set V"=w718:string, "error out"=w724:errorcluster)  [unwired: 8 in, 3 out]
          n431 = call "(Instrl) HVPS_2.vi"("Write Data"=w718, "error in (no error)"=w724, "CMD"=(Ctrl)_State_HVPS_CMD."Tx : Set V" ("State")) -> ("error out"=w722:errorcluster)  [unwired: 11 in, 5 out]
          n432 = while {
            shift-right: [FALSE] -> _
            shift-left: TRUE -> [w736]
            tunnel: w722 -> [_]
            tunnel: [w731] -> w721
            stop <- w732 stop-if-true
            n433 = global read "(Var) Get_HVPS_2.vi" "G2. Q Stop"() -> (w728:bool)
            n434 = local read "G2.Comm"() -> (w730:bool)
            n435 = call "경과 시간5"("Time Target (s)"=5.0, "Reset"=w736, "Auto Reset"=FALSE) -> ("Time has Elapsed"=w734:bool)  [unwired: 9 in, 7 out]
            n436 = Wait Until Next ms Multiple(millisecond multiple=u32 1 ("ms 배수")) -> ()  [unwired: 1 out]
            n437 = Compound Arithmetic op=OR ("복합 연산")(w730, w734, w728) -> (w732:bool)
            n438 = Compound Arithmetic op=OR ("복합 연산")(w730, w728) -> (w731:bool)
          }
        }
        n439 = global read "(Var) Get_HVPS_2.vi" "G2. Q Stop"() -> (w679:bool)
        n440 = case shown="거짓" w679 {
          tunnel: w689 -> [w698 _]
          tunnel: [w695 errorcluster {"status"=FALSE, "code"=0, "source"=""} ("에러 상수")] -> w680
          frame False {
            n441 = stacked-sequence {
              tunnel: w698 -> [_ _ _ _]
              tunnel: [w700 _ _ _] -> w696
              tunnel: [_ w705 _ _] -> w697
              frame #0 {
                w702 = 0.0  # Set mA
                # "0mA SET"
                n442 = call "(Sub) CMD Parsing_2.vi"("State"=(Ctrl)_State_Parcing."Set mA", "Set mA"=w702) -> ("CMD Set mA"=w701:string, "error out"=w704:errorcluster)  [unwired: 9 in, 3 out]
                n443 = call "(Instrl) HVPS_2.vi"("Write Data"=w701, "error in (no error)"=w704, "CMD"=(Ctrl)_State_HVPS_CMD."Tx : Set mA" ("State")) -> ("error out"=w700:errorcluster)  [unwired: 11 in, 5 out]
              }
              frame #1 {
                # "Power OFF"
                n444 = call "(Instrl) HVPS_2.vi"("CMD"=(Ctrl)_State_HVPS_CMD."Tx : OFF" ("State")) -> ("error out"=w705:errorcluster)  [unwired: 13 in, 5 out]
              }
              frame #2 {
                n445 = local write "G2_TEST END?"(TRUE ("G1_TEST END?")) -> ()
                n446 = local write "G2. Test  Status"(u16 5 ("Test END")) -> ()
                n447 = global write "(Var) Get_HVPS_2.vi" "G2. Start"(FALSE ("G2. Start")) -> ()
                n448 = global write "(Var) Get_HVPS_2.vi" "G2. Stop"(TRUE ("G2. Stop")) -> ()
              }
              frame #3 {
                n449 = property on="G2. Start Delay" class="DigNum (엄격한)"("DisabledEnum"=T7."Enabled" ("비활성화")) -> ()  [unwired: 2 in, 2 out]
                n450 = property on="Group2. Info" class="Str"("DisabledEnum"=T7."Enabled" ("비활성화")) -> ()  [unwired: 2 in, 2 out]
                n451 = property on="G2. Start Butten" class="Bool"("DisabledEnum"=T7."Enabled" ("비활성화")) -> ()  [unwired: 2 in, 2 out]
                n452 = property on="G2. Stop Butten" class="Bool"("DisabledEnum"=T7."Disabled and Grayed Out" ("비활성화")) -> ()  [unwired: 2 in, 2 out]
                n453 = property on="G2. Taget Voltage" class="DigNum (엄격한)"("DisabledEnum"=T7."Enabled" ("비활성화")) -> ()  [unwired: 2 in, 2 out]
                n454 = property on="G2. Current Limit" class="DigNum (엄격한)"("DisabledEnum"=T7."Enabled" ("비활성화")) -> ()  [unwired: 2 in, 2 out]
              }
            }
            n455 = Merge Errors(w696, w697) -> (w695:errorcluster)
          }
          frame True {
          }
        }
        n456 = flat-sequence {
          tunnel: [w694] -> w688
          tunnel: w680 -> [_]
          frame #0 {
            n457 = global read "(Var) Get_HVPS_2.vi" "G2. Q Stop"() -> (w691:bool)
            n458 = Select(t=(Ctrl)_State_Test_Manage."Quick Falling" ("State"), s=w691, f=(Ctrl)_State_Test_Manage."Idls" ("State")) -> (s? t:f=w694:T1)
          }
        }
      }
      frame "Quick Falling" {
        n459 = local write "G2. Test  Status"(u16 6 ("G1. Test  Status")) -> ()
        n460 = stacked-sequence {
          tunnel: [_ _ w760 _ _] -> w740
          tunnel: w747 -> [_ _ _ _ _]
          tunnel: [w749 _ _ _ _] -> w742
          tunnel: [_ w755 _ _ _] -> w741
          frame #0 {
            w751 = 0.0  # Set V
            # "0V SET"
            n461 = call "(Sub) CMD Parsing_2.vi"("Set V"=w751, "State"=(Ctrl)_State_Parcing."Set V") -> ("CMD Set V"=w750:string, "error out"=w753:errorcluster)  [unwired: 9 in, 3 out]
            n462 = call "(Instrl) HVPS_2.vi"("Write Data"=w750, "error in (no error)"=w753, "CMD"=(Ctrl)_State_HVPS_CMD."Tx : Set V" ("State")) -> ("error out"=w749:errorcluster)  [unwired: 11 in, 5 out]
          }
          frame #1 {
            w757 = 0.0  # Set mA
            # "0mA SET"
            n463 = call "(Sub) CMD Parsing_2.vi"("State"=(Ctrl)_State_Parcing."Set mA", "Set mA"=w757) -> ("CMD Set mA"=w756:string, "error out"=w759:errorcluster)  [unwired: 9 in, 3 out]
            n464 = call "(Instrl) HVPS_2.vi"("Write Data"=w756, "error in (no error)"=w759, "CMD"=(Ctrl)_State_HVPS_CMD."Tx : Set mA" ("State")) -> ("error out"=w755:errorcluster)  [unwired: 11 in, 5 out]
          }
          frame #2 {
            # "Power OFF"
            n465 = call "(Instrl) HVPS_2.vi"("CMD"=(Ctrl)_State_HVPS_CMD."Tx : OFF" ("State")) -> ("error out"=w760:errorcluster)  [unwired: 13 in, 5 out]
          }
          frame #3 {
            w765 = u16 6  # Shutdown
            n466 = local write "G2. Test  Status"(w765) -> ()
            n467 = local write "G2_TEST END?"(TRUE ("G1_TEST END?")) -> ()
            n468 = global write "(Var) Get_HVPS_2.vi" "G2. Start"(FALSE ("G2. Start")) -> ()
            n469 = global write "(Var) Get_HVPS_2.vi" "G2. Stop"(TRUE ("G2. Stop")) -> ()
          }
          frame #4 {
            n470 = property on="G2. Start Delay" class="DigNum (엄격한)"("DisabledEnum"=T7."Enabled" ("비활성화")) -> ()  [unwired: 2 in, 2 out]
            n471 = property on="Group2. Info" class="Str"("DisabledEnum"=T7."Enabled" ("비활성화")) -> ()  [unwired: 2 in, 2 out]
            n472 = property on="G2. Start Butten" class="Bool"("DisabledEnum"=T7."Enabled" ("비활성화")) -> ()  [unwired: 2 in, 2 out]
            n473 = property on="G2. Stop Butten" class="Bool"("DisabledEnum"=T7."Disabled and Grayed Out" ("비활성화")) -> ()  [unwired: 2 in, 2 out]
            n474 = property on="G2. Taget Voltage" class="DigNum (엄격한)"("DisabledEnum"=T7."Enabled" ("비활성화")) -> ()  [unwired: 2 in, 2 out]
            n475 = property on="G2. Current Limit" class="DigNum (엄격한)"("DisabledEnum"=T7."Enabled" ("비활성화")) -> ()  [unwired: 2 in, 2 out]
          }
        }
        n476 = Merge Errors(w742, w741, w740) -> (w739:errorcluster)
        n477 = local read "Exit ?"() -> (w746:bool)
        n478 = Select(t=(Ctrl)_State_Test_Manage."Close" ("State"), s=w746, f=(Ctrl)_State_Test_Manage."Idls" ("State")) -> (s? t:f=w745:T1)
      }
      frame "Close" {
        n479 = flat-sequence {
          tunnel: [w776] -> w773
          tunnel: w772 -> [_]
          frame #0 {
            n480 = call "(Instrl) HVPS_2.vi"("CMD"=(Ctrl)_State_HVPS_CMD."Close" ("State")) -> ("error out"=w776:errorcluster)  [unwired: 13 in, 5 out]
          }
        }
      }
    }
    "G2. State" <- w515
  }
  n481 = while "Group.3 HVPS Manager Loop" {
    shift-right: [w783] -> _
    shift-left: (Ctrl)_State_Test_Manage."Idls" ("State") -> [w784]
    tunnel: w1 -> [w780]
    tunnel: [w781] -> w8
    shift-right: [w778] -> _
    shift-left: _ -> [w779]
    stop <- w782 stop-if-true
    n482 = case shown="\"Run\"" w784 {
      tunnel: [w794 w830 w877 (Ctrl)_State_Test_Manage."Run" ("State") w953 w1010 (Ctrl)_State_Test_Manage."Close" ("State")] -> w783
      tunnel: [_ _ _ _ _ _ TRUE] -> w782
      tunnel: w780 -> [w798 w836 _ w900 w955 w1012 w1037]
      tunnel: [_ w832 _ _ w945 w1004 w1038] -> w781
      tunnel: w779 -> [_ _ w871 _ _ _ _]
      tunnel: [_ _ _ TRUE _ _ _] -> w778
      frame "Idls", Default {
        n483 = local read "G3_TEST END?"() -> (w787:bool)
        n484 = flat-sequence {
          tunnel: w798 -> [w821]
          tunnel: [w820] -> w800
          tunnel: [w821] -> w799
          tunnel: [w827] -> w793
          tunnel: w800 -> [w824]
          tunnel: w799 -> [w827]
          tunnel: [w822] -> w792
          frame #0 {
            n485 = global read "(Var) Get_HVPS_3.vi" "G3. Start"() -> (w820:bool)
          }
          frame #1 {
            n486 = local read "G3_TEST END?"() -> (w825:bool)
            n487 = Wait (ms)(milliseconds to wait=u32 300 ("대기 시간 (ms)")) -> ()  [unwired: 1 out]
            n488 = Select(t=FALSE, s=w825, f=w824) -> (s? t:f=w822:bool)
          }
        }
        n489 = case shown="거짓" w787 {
          frame False {
            w814 = 1  # Ready
            w815 = 0  # NOT Ready
            n490 = local read "G3.System"() -> (w818:bool)
            n491 = local read "G3.Comm"() -> (w819:bool)
            n492 = Compound Arithmetic op=AND(w819, w818, TRUE) -> (w816:bool)
            n493 = Select(t=w815, s=w816, f=w814) -> (s? t:f=w813:i32)
            n494 = local write "G3. Test  Status"(w813) -> ()
          }
          frame True {
          }
        }
        n495 = local read "G3.Comm"() -> (w785:bool)
        n496 = case shown="거짓" w785 {
          tunnel: w793 -> [w802 w805]
          tunnel: [w802 w808] -> w786
          frame False {
          }
          frame True {
            w806 = u16 50001  # Port
            w807 = "192.168.10.63"  # IP
            n497 = call "(Instrl) HVPS_3.vi"("error in (no error)"=w805, "CMD"=(Ctrl)_State_HVPS_CMD."Close" ("State")) -> ("error out"=w803:errorcluster)  [unwired: 12 in, 5 out]
            n498 = call "(Instrl) HVPS_3.vi"("IP"=w807, "Port"=w806, "error in (no error)"=w803, "CMD"=(Ctrl)_State_HVPS_CMD."Open" ("State")) -> ("error out"=w808:errorcluster)  [unwired: 10 in, 5 out]
          }
        }
        n499 = case shown="에러" w786 {
          selector: w786 -> [w810 w812]
          tunnel: [w810 w812] -> w789
          frame No Error {
          }
          frame Error {
            n500 = global read "(Var) Get_HVPS_3.vi" "G3. Stop"() -> (w811:bool)
            n501 = local write "G3_TEST END?"(w811) -> ()
          }
        }
        n502 = Select(t=(Ctrl)_State_Test_Manage."Run Init" ("State"), s=w792, f=(Ctrl)_State_Test_Manage."Idls" ("State")) -> (s? t:f=w791:T1)
        n503 = Select(t=(Ctrl)_State_Test_Manage."Idls" ("State"), s=w789, f=w791) -> (s? t:f=w788:T1)
        n504 = local read "Exit ?"() -> (w797:bool)
        n505 = Select(t=(Ctrl)_State_Test_Manage."Close" ("State"), s=w797, f=w788) -> (s? t:f=w794:T1)
      }
      frame "Run Init" {
        n506 = flat-sequence {
          tunnel: w836 -> [w855]
          tunnel: [w855] -> w835
          tunnel: [w863] -> w833
          tunnel: w835 -> [w863]
          frame #0 {
            w852 = 0.0 ("G1. KV")
            n507 = global write "(Var) Get_HVPS_3.vi" "G3. mA"(w852) -> ()
            n508 = global write "(Var) Get_HVPS_3.vi" "G3. KV"(w852) -> ()
            n509 = call "(Sub) Falling Step.vi"("State"=T9."G3. Reset") -> ()  [unwired: 7 in, 4 out]
            n510 = property on="G3. Current Graph" class="WFChart (엄격한)"("History Data"=T10 [] ("히스토리 데이터")) -> ()  [unwired: 2 in, 2 out]
            n511 = property on="G3. Voltage Graph" class="WFChart (엄격한)"("History Data"=dbl[] [] ("히스토리 데이터")) -> ()  [unwired: 2 in, 2 out]
          }
          frame #1 {
            n512 = property on="G3. Start Delay" class="DigNum (엄격한)"("DisabledEnum"=T7."Disabled and Grayed Out" ("비활성화")) -> ()  [unwired: 2 in, 2 out]
            n513 = property on="Group3. Info" class="Str"("DisabledEnum"=T7."Disabled and Grayed Out" ("비활성화")) -> ()  [unwired: 2 in, 2 out]
            n514 = property on="G3. Delay" class="DigNum (엄격한)"("Visible"=TRUE ("보이기")) -> ()  [unwired: 2 in, 2 out]
            n515 = property on="G3. Start Butten" class="Bool"("DisabledEnum"=T7."Disabled and Grayed Out" ("비활성화")) -> ()  [unwired: 2 in, 2 out]
            n516 = property on="G3. Stop Butten" class="Bool"("DisabledEnum"=T7."Enabled" ("비활성화")) -> ()  [unwired: 2 in, 2 out]
            n517 = property on="G3. Taget Voltage" class="DigNum (엄격한)"("DisabledEnum"=T7."Disabled and Grayed Out" ("비활성화")) -> ()  [unwired: 2 in, 2 out]
            n518 = property on="G3. Current Limit" class="DigNum (엄격한)"("DisabledEnum"=T7."Disabled and Grayed Out" ("비활성화")) -> ()  [unwired: 2 in, 2 out]
          }
        }
        n519 = local write "G3. Test  Status"(u16 7 ("G1. Test  Status")) -> ()
        n520 = Get Date/Time In Seconds() -> (seconds since 1Jan1904=w834:timestamp)
        n521 = while {
          tunnel: w833 -> [w850]
          tunnel: [w850] -> w828
          tunnel: w834 -> [w849]
          stop <- w845 stop-if-true
          n522 = Get Date/Time In Seconds() -> (seconds since 1Jan1904=w848:timestamp)
          n523 = local read "Start Delay"() -> (w844:dbl)
          n524 = Subtract(x=w848, y=w849) -> (x-y=w843:dbl)
          n525 = global read "(Var) Get_HVPS_3.vi" "G3. Stop"() -> (w841:bool)
          n526 = Greater Or Equal?(x=w843, y=w844) -> (x >= y?=w847:bool)
          n527 = Subtract(x=w844, y=w843) -> (x-y=→"G3. Delay":dbl)
          n528 = Or(x=w847, y=w841) -> (x .or. y?=w845:bool)
          n529 = Wait (ms)(milliseconds to wait=u32 1 ("대기 시간 (ms)")) -> ()  [unwired: 1 out]
        }
        n530 = flat-sequence {
          tunnel: [w838] -> w830
          tunnel: w828 -> [_]
          frame #0 {
            n531 = global read "(Var) Get_HVPS_3.vi" "G3. Stop"() -> (w837:bool)
            n532 = Select(t=(Ctrl)_State_Test_Manage."Falling" ("State"), s=w837, f=(Ctrl)_State_Test_Manage."Rising" ("State")) -> (s? t:f=w838:T1)
          }
        }
        n533 = property on="G3. Delay" class="DigNum (엄격한)"(error in=w828, "Visible"=FALSE ("보이기")) -> (error out=w832:errorcluster)  [unwired: 1 in, 1 out]
      }
      frame "Run" {
        # "Limit 값 넘으면, Quick Stop\nQuick Stop 버튼 누르면, Quick Stop\nExit 버튼 누르면, Quick Stop\nStop 버튼 누르면, Stop"
        n534 = local read "G3.Comm"() -> (w881:bool)
        n535 = local write "G3. Test  Status"(u16 2 ("G1. Test  Status")) -> ()
        n536 = local read "G3. Current Limit"() -> (w875:dbl)
        n537 = call "경과 시간10"("Reset"=w871, "Auto Reset"=FALSE) -> ("Elapsed Time (s)"=w872:dbl)  [unwired: 10 in, 7 out]
        n538 = global read "(Var) Get_HVPS_3.vi" "G3. mA"() -> (w864:dbl)
        n539 = local read "G3. Target Time"() -> (w873:dbl)
        n540 = local write "G3. Time"(w872) -> ()
        n541 = Greater Or Equal?(x=w864, y=w875) -> (x >= y?=w887:bool)
        n542 = Wait Until Next ms Multiple(millisecond multiple=u32 300 ("대기 시간 (ms)")) -> ()  [unwired: 1 out]
        n543 = Greater Or Equal?(x=w872, y=w873) -> (x >= y?=w868:bool)
        n544 = Select(t=(Ctrl)_State_Test_Manage."Idls" ("State"), s=w881, f=(Ctrl)_State_Test_Manage."Run" ("State")) -> (s? t:f=w879:T1)
        n545 = global read "(Var) Get_HVPS_3.vi" "G3. Start"() -> (w866:bool)
        n546 = Select(t=(Ctrl)_State_Test_Manage."Quick Falling" ("State"), s=w887, f=w879) -> (s? t:f=w885:T1)
        n547 = Select(t=w885, s=w866, f=(Ctrl)_State_Test_Manage."Falling" ("State")) -> (s? t:f=w869:T1)
        n548 = global read "(Var) Get_HVPS_3.vi" "G3. Q Stop"() -> (w865:bool)
        n549 = Select(t=(Ctrl)_State_Test_Manage."Falling" ("State"), s=w868, f=w869) -> (s? t:f=w867:T1)
        n550 = Select(t=(Ctrl)_State_Test_Manage."Quick Falling" ("State"), s=w865, f=w867) -> (s? t:f=w877:T1)
      }
      frame "Rising" {
        n551 = stacked-sequence {
          tunnel: w900 -> [_ _ _ _]
          tunnel: [w923 _ _ _] -> w898
          tunnel: [_ w929 _ _] -> w897
          tunnel: [_ _ w934 _] -> w896
          tunnel: [_ _ _ w939] -> w895
          frame #0 {
            w926 = 0.0  # Set V
            # "0V SET"
            n552 = call "(Sub) CMD Parsing_3.vi"("Set V"=w926, "State"=(Ctrl)_State_Parcing."Set V") -> ("CMD Set V"=w922:string, "error out"=w927:errorcluster)  [unwired: 9 in, 3 out]
            n553 = call "(Instrl) HVPS_3.vi"("Write Data"=w922, "error in (no error)"=w927, "CMD"=(Ctrl)_State_HVPS_CMD."Tx : Set V" ("State")) -> ("error out"=w923:errorcluster)  [unwired: 11 in, 5 out]
          }
          frame #1 {
            w931 = 0.0  # Set mA
            # "0mA SET"
            n554 = call "(Sub) CMD Parsing_3.vi"("State"=(Ctrl)_State_Parcing."Set mA", "Set mA"=w931) -> ("CMD Set mA"=w930:string, "error out"=w933:errorcluster)  [unwired: 9 in, 3 out]
            n555 = call "(Instrl) HVPS_3.vi"("Write Data"=w930, "error in (no error)"=w933, "CMD"=(Ctrl)_State_HVPS_CMD."Tx : Set mA" ("State")) -> ("error out"=w929:errorcluster)  [unwired: 11 in, 5 out]
          }
          frame #2 {
            # "Power ON"
            n556 = call "(Instrl) HVPS_3.vi"("CMD"=(Ctrl)_State_HVPS_CMD."Tx : ON" ("State")) -> ("error out"=w934:errorcluster)  [unwired: 13 in, 5 out]
          }
          frame #3 {
            # "mA SET"
            n557 = local read "G3. Current Limit"() -> (w936:dbl)
            n558 = call "(Sub) CMD Parsing_3.vi"("State"=(Ctrl)_State_Parcing."Set mA", "Set mA"=w936) -> ("CMD Set mA"=w937:string, "error out"=w941:errorcluster)  [unwired: 9 in, 3 out]
            n559 = call "(Instrl) HVPS_3.vi"("Write Data"=w937, "error in (no error)"=w941, "CMD"=(Ctrl)_State_HVPS_CMD."Tx : Set mA" ("State")) -> ("error out"=w939:errorcluster)  [unwired: 11 in, 5 out]
          }
        }
        n560 = local write "G3. Test  Status"(u16 3 ("G1. Test  Status")) -> ()
        n561 = local read "G3. Taget Voltage"() -> (w892:dbl)
        n562 = Merge Errors(w898, w897, w896, w895) -> (w894:errorcluster)
        n563 = call "(Sub) Power Sweep.vi"("Taget Voltage"=w892) -> ("ON Sweep"=w891:dbl[])  [unwired: 8 in, 2 out]
        n564 = case shown="에러 없음" w894 {
          selector: w894 -> [w902 _]
          tunnel: w891 -> [w903 w921]
          tunnel: [w901 w921] -> w888
          frame No Error {
            n565 = for {
              tunnel: w902 -> [w911]
              tunnel: w903 -> [w904] mode=indexing
              tunnel: [w904] -> w901 mode=indexing
              stop <- w907 stop-if-true
              n566 = call "(Sub) CMD Parsing_3.vi"("Set V"=w904, "State"=(Ctrl)_State_Parcing."Set V", "error in (no error)"=w911) -> ("CMD Set V"=w905:string, "error out"=w910:errorcluster)  [unwired: 8 in, 3 out]
              n567 = call "(Instrl) HVPS_3.vi"("Write Data"=w905, "error in (no error)"=w910, "CMD"=(Ctrl)_State_HVPS_CMD."Tx : Set V" ("State")) -> ("error out"=w908:errorcluster)  [unwired: 11 in, 5 out]
              n568 = while {
                shift-right: [FALSE] -> _
                shift-left: TRUE -> [w919]
                tunnel: w908 -> [_]
                tunnel: [w913] -> w907
                stop <- w915 stop-if-true
                n569 = global read "(Var) Get_HVPS_3.vi" "G3. Stop"() -> (w913:bool)
                n570 = call "경과 시간6"("Time Target (s)"=5.0, "Reset"=w919, "Auto Reset"=FALSE) -> ("Time has Elapsed"=w917:bool)  [unwired: 9 in, 7 out]
                n571 = Wait Until Next ms Multiple(millisecond multiple=u32 1 ("ms 배수")) -> ()  [unwired: 1 out]
                n572 = Or(x=w917, y=w913) -> (x .or. y?=w915:bool)
              }
            }
          }
          frame Error {
          }
        }
        n573 = call "(Sub) Falling Step.vi"("State"=T9."G3. Save", "G3. Rising Step"=w888) -> ()  [unwired: 6 in, 4 out]
      }
      frame "Falling" {
        n574 = local write "G3. Test  Status"(u16 4 ("G1. Test  Status")) -> ()
        n575 = call "(Sub) Falling Step.vi"("State"=T9."G3. Load") -> ("G3. Falling Step"=w942:dbl[])  [unwired: 7 in, 3 out]
        n576 = Reverse 1D Array(array=w942) -> (reversed array=w950:dbl[])
        n577 = Build Array (concatenate)(w950, 0.0) -> (w947:dbl[])
        n578 = Delete From Array(array=w947, length=1 ("길이"), index=0 ("인덱스")) -> (array with subset deleted=w946:dbl[])  [unwired: 1 out]
        n579 = for {
          tunnel: w955 -> [w967]
          tunnel: w946 -> [w968] mode=indexing
          tunnel: [errorcluster {"status"=FALSE, "code"=0, "source"=""} ("에러 상수")] -> w954
          stop <- w963 stop-if-true
          n580 = call "(Sub) CMD Parsing_3.vi"("Set V"=w968, "State"=(Ctrl)_State_Parcing."Set V", "error in (no error)"=w967) -> ("CMD Set V"=w960:string, "error out"=w966:errorcluster)  [unwired: 8 in, 3 out]
          n581 = call "(Instrl) HVPS_3.vi"("Write Data"=w960, "error in (no error)"=w966, "CMD"=(Ctrl)_State_HVPS_CMD."Tx : Set V" ("State")) -> ("error out"=w964:errorcluster)  [unwired: 11 in, 5 out]
          n582 = while {
            shift-right: [FALSE] -> _
            shift-left: TRUE -> [w978]
            tunnel: w964 -> [_]
            tunnel: [w973] -> w963
            stop <- w974 stop-if-true
            n583 = global read "(Var) Get_HVPS_3.vi" "G3. Q Stop"() -> (w970:bool)
            n584 = local read "G3.Comm"() -> (w972:bool)
            n585 = call "경과 시간7"("Time Target (s)"=5.0, "Reset"=w978, "Auto Reset"=FALSE) -> ("Time has Elapsed"=w976:bool)  [unwired: 9 in, 7 out]
            n586 = Wait Until Next ms Multiple(millisecond multiple=u32 1 ("ms 배수")) -> ()  [unwired: 1 out]
            n587 = Compound Arithmetic op=OR ("복합 연산")(w972, w976, w970) -> (w974:bool)
            n588 = Compound Arithmetic op=OR ("복합 연산")(w972, w970) -> (w973:bool)
          }
        }
        n589 = global read "(Var) Get_HVPS_3.vi" "G3. Q Stop"() -> (w944:bool)
        n590 = case shown="거짓" w944 {
          tunnel: w954 -> [w983 _]
          tunnel: [w980 errorcluster {"status"=FALSE, "code"=0, "source"=""} ("에러 상수")] -> w945
          frame False {
            n591 = stacked-sequence {
              tunnel: w983 -> [_ _ _ _]
              tunnel: [w985 _ _ _] -> w981
              tunnel: [_ w990 _ _] -> w982
              frame #0 {
                w987 = 0.0  # Set mA
                # "0mA SET"
                n592 = call "(Sub) CMD Parsing_3.vi"("State"=(Ctrl)_State_Parcing."Set mA", "Set mA"=w987) -> ("CMD Set mA"=w986:string, "error out"=w989:errorcluster)  [unwired: 9 in, 3 out]
                n593 = call "(Instrl) HVPS_3.vi"("Write Data"=w986, "error in (no error)"=w989, "CMD"=(Ctrl)_State_HVPS_CMD."Tx : Set mA" ("State")) -> ("error out"=w985:errorcluster)  [unwired: 11 in, 5 out]
              }
              frame #1 {
                # "Power OFF"
                n594 = call "(Instrl) HVPS_3.vi"("CMD"=(Ctrl)_State_HVPS_CMD."Tx : OFF" ("State")) -> ("error out"=w990:errorcluster)  [unwired: 13 in, 5 out]
              }
              frame #2 {
                n595 = local write "G3_TEST END?"(TRUE ("G1_TEST END?")) -> ()
                n596 = local write "G3. Test  Status"(u16 5 ("Test END")) -> ()
                n597 = global write "(Var) Get_HVPS_3.vi" "G3. Stop"(TRUE) -> ()
                n598 = global write "(Var) Get_HVPS_3.vi" "G3. Start"(FALSE) -> ()
              }
              frame #3 {
                n599 = property on="G3. Start Butten" class="Bool"("DisabledEnum"=T7."Enabled" ("비활성화")) -> ()  [unwired: 2 in, 2 out]
                n600 = property on="G3. Stop Butten" class="Bool"("DisabledEnum"=T7."Disabled and Grayed Out" ("비활성화")) -> ()  [unwired: 2 in, 2 out]
                n601 = property on="G3. Taget Voltage" class="DigNum (엄격한)"("DisabledEnum"=T7."Enabled" ("비활성화")) -> ()  [unwired: 2 in, 2 out]
                n602 = property on="G3. Current Limit" class="DigNum (엄격한)"("DisabledEnum"=T7."Enabled" ("비활성화")) -> ()  [unwired: 2 in, 2 out]
                n603 = property on="G3. Start Delay" class="DigNum (엄격한)"("DisabledEnum"=T7."Enabled" ("비활성화")) -> ()  [unwired: 2 in, 2 out]
                n604 = property on="Group3. Info" class="Str"("DisabledEnum"=T7."Enabled" ("비활성화")) -> ()  [unwired: 2 in, 2 out]
              }
            }
            n605 = Merge Errors(w981, w982) -> (w980:errorcluster)
          }
          frame True {
          }
        }
        n606 = flat-sequence {
          tunnel: [w959] -> w953
          tunnel: w945 -> [_]
          frame #0 {
            n607 = global read "(Var) Get_HVPS_3.vi" "G3. Q Stop"() -> (w956:bool)
            n608 = Select(t=(Ctrl)_State_Test_Manage."Quick Falling" ("State"), s=w956, f=(Ctrl)_State_Test_Manage."Idls" ("State")) -> (s? t:f=w959:T1)
          }
        }
      }
      frame "Quick Falling" {
        n609 = local write "G3. Test  Status"(u16 6 ("G1. Test  Status")) -> ()
        n610 = stacked-sequence {
          tunnel: [_ _ w1025 _ _] -> w1005
          tunnel: w1012 -> [_ _ _ _ _]
          tunnel: [w1014 _ _ _ _] -> w1007
          tunnel: [_ w1020 _ _ _] -> w1006
          frame #0 {
            w1016 = 0.0  # Set V
            # "0V SET"
            n611 = call "(Sub) CMD Parsing_3.vi"("Set V"=w1016, "State"=(Ctrl)_State_Parcing."Set V") -> ("CMD Set V"=w1015:string, "error out"=w1018:errorcluster)  [unwired: 9 in, 3 out]
            n612 = call "(Instrl) HVPS_3.vi"("Write Data"=w1015, "error in (no error)"=w1018, "CMD"=(Ctrl)_State_HVPS_CMD."Tx : Set V" ("State")) -> ("error out"=w1014:errorcluster)  [unwired: 11 in, 5 out]
          }
          frame #1 {
            w1022 = 0.0  # Set mA
            # "0mA SET"
            n613 = call "(Sub) CMD Parsing_3.vi"("State"=(Ctrl)_State_Parcing."Set mA", "Set mA"=w1022) -> ("CMD Set mA"=w1021:string, "error out"=w1024:errorcluster)  [unwired: 9 in, 3 out]
            n614 = call "(Instrl) HVPS_3.vi"("Write Data"=w1021, "error in (no error)"=w1024, "CMD"=(Ctrl)_State_HVPS_CMD."Tx : Set mA" ("State")) -> ("error out"=w1020:errorcluster)  [unwired: 11 in, 5 out]
          }
          frame #2 {
            # "Power OFF"
            n615 = call "(Instrl) HVPS_3.vi"("CMD"=(Ctrl)_State_HVPS_CMD."Tx : OFF" ("State")) -> ("error out"=w1025:errorcluster)  [unwired: 13 in, 5 out]
          }
          frame #3 {
            w1030 = u16 6  # Shutdown
            n616 = local write "G3. Test  Status"(w1030) -> ()
            n617 = local write "G3_TEST END?"(TRUE ("G1_TEST END?")) -> ()
            n618 = global write "(Var) Get_HVPS_3.vi" "G3. Start"(FALSE) -> ()
            n619 = global write "(Var) Get_HVPS_3.vi" "G3. Stop"(TRUE) -> ()
          }
          frame #4 {
            n620 = property on="G3. Start Delay" class="DigNum (엄격한)"("DisabledEnum"=T7."Enabled" ("비활성화")) -> ()  [unwired: 2 in, 2 out]
            n621 = property on="Group3. Info" class="Str"("DisabledEnum"=T7."Enabled" ("비활성화")) -> ()  [unwired: 2 in, 2 out]
            n622 = property on="G3. Start Butten" class="Bool"("DisabledEnum"=T7."Enabled" ("비활성화")) -> ()  [unwired: 2 in, 2 out]
            n623 = property on="G3. Stop Butten" class="Bool"("DisabledEnum"=T7."Disabled and Grayed Out" ("비활성화")) -> ()  [unwired: 2 in, 2 out]
            n624 = property on="G3. Taget Voltage" class="DigNum (엄격한)"("DisabledEnum"=T7."Enabled" ("비활성화")) -> ()  [unwired: 2 in, 2 out]
            n625 = property on="G3. Current Limit" class="DigNum (엄격한)"("DisabledEnum"=T7."Enabled" ("비활성화")) -> ()  [unwired: 2 in, 2 out]
          }
        }
        n626 = Merge Errors(w1007, w1006, w1005) -> (w1004:errorcluster)
        n627 = local read "Exit ?"() -> (w1011:bool)
        n628 = Select(t=(Ctrl)_State_Test_Manage."Close" ("State"), s=w1011, f=(Ctrl)_State_Test_Manage."Idls" ("State")) -> (s? t:f=w1010:T1)
      }
      frame "Close" {
        n629 = flat-sequence {
          tunnel: [w1041] -> w1038
          tunnel: w1037 -> [_]
          frame #0 {
            n630 = call "(Instrl) HVPS_3.vi"("CMD"=(Ctrl)_State_HVPS_CMD."Close" ("State")) -> ("error out"=w1041:errorcluster)  [unwired: 13 in, 5 out]
          }
        }
      }
    }
    "G3. State" <- w784
  }
  n631 = while "State Display Loop" {
    tunnel: w1 -> [_]
    stop <- w1043 stop-if-true
    n632 = stacked-sequence {
      frame #0 {
        # "State Updata"
        n633 = global read "(Var) Chamber.vi" "Chamber Temp"() -> (→"Chamber Temp":dbl)
        n634 = global read "(Var) Get_HVPS_1.vi" "G1. Read Mode"() -> (w1057:string)
        n635 = global read "(Var) Get_HVPS_2.vi" "G2. Read Mode"() -> (w1054:string)
        n636 = global read "(Var) Get_HVPS_3.vi" "G3. Read Mode"() -> (w1051:string)
        n637 = global read "(Var) Get_HVPS_1.vi" "G1. Read State"() -> (w1059:string)
        n638 = global read "(Var) Get_HVPS_2.vi" "G2. Read State"() -> (w1056:string)
        n639 = global read "(Var) Get_HVPS_3.vi" "G3. Read State"() -> (w1053:string)
        n640 = global read "(Var) Chamber.vi" "Target Temp"() -> (w1046:u16)
        n641 = global read "(Var) Get_HVPS_1.vi" "G1. Error ?"() -> (w1050:bool)
        n642 = global read "(Var) Get_HVPS_2.vi" "G2. Error ?"() -> (w1049:bool)
        n643 = global read "(Var) Get_HVPS_3.vi" "G3. Error ?"() -> (w1048:bool)
        n644 = global read "(Var) Get_HVPS_1.vi" "G1. Read HV"() -> (w1058:string)
        n645 = global read "(Var) Get_HVPS_2.vi" "G2. Read HV"() -> (w1055:string)
        n646 = global read "(Var) Get_HVPS_3.vi" "G3. Read HV"() -> (w1052:string)
        n647 = global read "(Var) Chamber.vi" "Run ?"() -> (w1045:bool)
        n648 = local write "Chamber"(w1045) -> ()
        n649 = local write "Target Temp"(w1046) -> ()
        n650 = local write "G1.Comm"(w1050) -> ()
        n651 = local write "G2.Comm"(w1049) -> ()
        n652 = local write "G3.Comm"(w1048) -> ()
        n653 = call "(Sub) System State Check.vi"("Read  Mode"=w1057, "Read HV State"=w1058, "Read System State"=w1059) -> ("시스템 비정상?"=w1064:bool, "Out System State"=w1065:T3)  [unwired: 6 in, 1 out]
        n654 = call "(Sub) System State Check.vi"("Read  Mode"=w1054, "Read HV State"=w1055, "Read System State"=w1056) -> ("시스템 비정상?"=w1060:bool, "Out System State"=w1061:T3)  [unwired: 6 in, 1 out]
        n655 = call "(Sub) System State Check.vi"("Read  Mode"=w1051, "Read HV State"=w1052, "Read System State"=w1053) -> ("시스템 비정상?"=w1062:bool, "Out System State"=w1063:T3)  [unwired: 6 in, 1 out]
        n656 = local write "G1.System"(w1064) -> ()
        n657 = local write "G1 System State"(w1065) -> ()
        n658 = local write "G2.System"(w1060) -> ()
        n659 = local write "G2 System State"(w1061) -> ()
        n660 = local write "G3 System State"(w1063) -> ()
        n661 = local write "G3.System"(w1062) -> ()
      }
      frame #1 {
        # "Butten Disable & Enable"
        n662 = global read "(Var) Get_HVPS_1.vi" "G1. Start"() -> (w1068:bool)
        n663 = global read "(Var) Get_HVPS_2.vi" "G2. Start"() -> (w1067:bool)
        n664 = global read "(Var) Get_HVPS_3.vi" "G3. Start"() -> (w1066:bool)
        n665 = case shown="거짓" w1068 {
          frame False {
            n666 = local read "G1. Test  Status"() -> (w1104:u16)
            n667 = Equal To 0?(x=w1104) -> (x = 0?=w1108:bool)
            n668 = Equal?(x=w1104, y=u16 1) -> (x = y?=w1107:bool)
            n669 = Equal?(x=w1104, y=u16 5) -> (x = y?=w1103:bool)
            n670 = Equal?(x=w1104, y=u16 6) -> (x = y?=w1102:bool)
            n671 = Compound Arithmetic op=OR ("복합 연산")(w1108, w1107, w1103, w1102) -> (w1101:bool)
            n672 = case shown="참" w1101 {
              frame False {
              }
              frame True {
                n673 = local read "G1.System"() -> (w1111:bool)
                n674 = local read "G1.Comm"() -> (w1112:bool)
                n675 = And(x=w1112, y=w1111) -> (x .and. y?=w1110:bool)
                n676 = case shown="거짓" w1110 {
                  frame False {
                    n677 = property on="G1. Start Butten" class="Bool"() -> ("DisabledEnum"=w1113:T7)  [unwired: 2 in, 2 out]
                    n678 = case shown="\"Disabled and Grayed Out\", 기본" w1113 {
                      frame "Enabled" {
                      }
                      frame "Disabled and Grayed Out", Default {
                        n679 = property on="G1. Start Butten" class="Bool"("DisabledEnum"=T7."Enabled" ("비활성화")) -> ()  [unwired: 2 in, 2 out]
                      }
                    }
                  }
                  frame True {
                    n680 = property on="G1. Start Butten" class="Bool"() -> ("DisabledEnum"=w1115:T7)  [unwired: 2 in, 2 out]
                    n681 = case shown="\"Enabled\", 기본" w1115 {
                      frame "Enabled", Default {
                        n682 = property on="G1. Start Butten" class="Bool"("DisabledEnum"=T7."Disabled and Grayed Out" ("비활성화")) -> ()  [unwired: 2 in, 2 out]
                      }
                      frame "Disabled and Grayed Out" {
                      }
                    }
                  }
                }
              }
            }
          }
          frame True {
          }
        }
        n683 = case shown="거짓" w1067 {
          frame False {
            n684 = local read "G2. Test  Status"() -> (w1088:u16)
            n685 = Equal To 0?(x=w1088) -> (x = 0?=w1092:bool)
            n686 = Equal?(x=w1088, y=u16 1) -> (x = y?=w1091:bool)
            n687 = Equal?(x=w1088, y=u16 5) -> (x = y?=w1087:bool)
            n688 = Equal?(x=w1088, y=u16 6) -> (x = y?=w1086:bool)
            n689 = Compound Arithmetic op=OR ("복합 연산")(w1092, w1091, w1087, w1086) -> (w1085:bool)
            n690 = case shown="참" w1085 {
              frame False {
              }
              frame True {
                n691 = local read "G2.System"() -> (w1095:bool)
                n692 = local read "G2.Comm"() -> (w1096:bool)
                n693 = And(x=w1096, y=w1095) -> (x .and. y?=w1094:bool)
                n694 = case shown="거짓" w1094 {
                  frame False {
                    n695 = property on="G2. Start Butten" class="Bool"() -> ("DisabledEnum"=w1097:T7)  [unwired: 2 in, 2 out]
                    n696 = case shown="\"Disabled and Grayed Out\", 기본" w1097 {
                      frame "Enabled" {
                      }
                      frame "Disabled and Grayed Out", Default {
                        n697 = property on="G2. Start Butten" class="Bool"("DisabledEnum"=T7."Enabled" ("비활성화")) -> ()  [unwired: 2 in, 2 out]
                      }
                    }
                  }
                  frame True {
                    n698 = property on="G2. Start Butten" class="Bool"() -> ("DisabledEnum"=w1099:T7)  [unwired: 2 in, 2 out]
                    n699 = case shown="\"Enabled\", 기본" w1099 {
                      frame "Enabled", Default {
                        n700 = property on="G2. Start Butten" class="Bool"("DisabledEnum"=T7."Disabled and Grayed Out" ("비활성화")) -> ()  [unwired: 2 in, 2 out]
                      }
                      frame "Disabled and Grayed Out" {
                      }
                    }
                  }
                }
              }
            }
          }
          frame True {
          }
        }
        n701 = case shown="거짓" w1066 {
          frame False {
            n702 = local read "G3. Test  Status"() -> (w1072:u16)
            n703 = Equal To 0?(x=w1072) -> (x = 0?=w1076:bool)
            n704 = Equal?(x=w1072, y=u16 1) -> (x = y?=w1075:bool)
            n705 = Equal?(x=w1072, y=u16 5) -> (x = y?=w1071:bool)
            n706 = Equal?(x=w1072, y=u16 6) -> (x = y?=w1070:bool)
            n707 = Compound Arithmetic op=OR ("복합 연산")(w1076, w1075, w1071, w1070) -> (w1069:bool)
            n708 = case shown="참" w1069 {
              frame False {
              }
              frame True {
                n709 = local read "G3.System"() -> (w1079:bool)
                n710 = local read "G3.Comm"() -> (w1080:bool)
                n711 = And(x=w1080, y=w1079) -> (x .and. y?=w1078:bool)
                n712 = case shown="거짓" w1078 {
                  frame False {
                    n713 = property on="G3. Start Butten" class="Bool"() -> ("DisabledEnum"=w1081:T7)  [unwired: 2 in, 2 out]
                    n714 = case shown="\"Disabled and Grayed Out\", 기본" w1081 {
                      frame "Enabled" {
                      }
                      frame "Disabled and Grayed Out", Default {
                        n715 = property on="G3. Start Butten" class="Bool"("DisabledEnum"=T7."Enabled" ("비활성화")) -> ()  [unwired: 2 in, 2 out]
                      }
                    }
                  }
                  frame True {
                    n716 = property on="G3. Start Butten" class="Bool"() -> ("DisabledEnum"=w1083:T7)  [unwired: 2 in, 2 out]
                    n717 = case shown="\"Enabled\", 기본" w1083 {
                      frame "Enabled", Default {
                        n718 = property on="G3. Start Butten" class="Bool"("DisabledEnum"=T7."Disabled and Grayed Out" ("비활성화")) -> ()  [unwired: 2 in, 2 out]
                      }
                      frame "Disabled and Grayed Out" {
                      }
                    }
                  }
                }
              }
            }
          }
          frame True {
          }
        }
      }
    }
    n719 = Wait Until Next ms Multiple(millisecond multiple=u32 500 ("대기 시간 (ms)")) -> ()  [unwired: 1 out]
    n720 = local read "Exit ?"() -> (w1043:bool)
  }
  n721 = while {
    tunnel: w1 -> [w1118]
    tunnel: [w1117] -> w19
    stop <- w1119 stop-if-true
    n722 = event shown="[5] \"Chamber\": 값 변경" {
      selector: _ -> [_ _ _ _ _ _ _ _ _ _ _ _ _ _ _ _ _]
      dyn-events: _ -> [_ _ _ _ _ _ _ _ _ _ _ _ _ _ _ _ _]
      timeout: _ -> [_ _ _ _ _ _ _ _ _ _ _ _ _ _ _ _ _]
      tunnel: [_ _ _ _ _ _ _ _ _ _ _ _ _ _ _ w1263 w1271] -> w1119
      tunnel: w1118 -> [_ _ _ _ _ _ w1214 w1219 w1224 w1229 w1233 w1237 _ _ _ _ _]
      tunnel: [_ _ _ _ _ _ _ _ _ _ _ _ _ _ _ errorcluster {"status"=FALSE, "code"=0, "source"=""} ("에러 상수") errorcluster {"status"=FALSE, "code"=0, "source"=""} ("에러 상수")] -> w1117
      event Timeout {
        n723 = event-data() -> ()  [unwired: 1 in, 3 out]
      }
      event "Radio_TAB": Value Change {
        n724 = event-data() -> ("NewVal"=w1120:enum32{"Home", "Manual Mode"})  [unwired: 1 in]
        n725 = case shown="\"Manual Mode\"" w1120 {
          frame "Home", Default {
            n726 = local write "탭 컨트롤"(enum32{"Display", "Manual Mode", "State"}."Display" ("탭 컨트롤")) -> ()
          }
          frame "Manual Mode" {
            n727 = local write "탭 컨트롤"(enum32{"Display", "Manual Mode", "State"}."Manual Mode" ("탭 컨트롤")) -> ()
          }
        }
      }
      event "Group.1 Manual": Value Change {
        n728 = event-data() -> ("NewVal"=w1125:T2)  [unwired: 1 in, 5 out]
        n729 = Unbundle(w1125) -> ("Bool_HV ON"=w1133:bool, "Bool_HV OFF"=w1132:bool, "Bool_Set V"=w1131:bool, "Bool_Set mA"=w1130:bool, "Bool_Get V"=w1129:bool, "Bool_Get mA"=w1128:bool, "Set V"=w1124:u16, "Set mA"=w1123:u16)
        n730 = Build Array(w1133, w1132, w1131, w1130, w1129, w1128) -> (w1127:bool[])
        n731 = Boolean Array To Number(Boolean array=w1127) -> (number=w1126:u32)
        n732 = case shown="4" w1126 {
          tunnel: w1124 -> [_ _ _ w1137 _ _ _]
          tunnel: w1123 -> [_ _ _ _ w1142 _ _]
          frame 0, Default {
          }
          frame 1 {
            # "HV ON"
            n733 = call "(Instrl) HVPS_1.vi"("CMD"=(Ctrl)_State_HVPS_CMD."Tx : ON" ("State")) -> ()  [unwired: 13 in, 6 out]
          }
          frame 2 {
            # "HV OFF"
            n734 = call "(Instrl) HVPS_1.vi"("CMD"=(Ctrl)_State_HVPS_CMD."Tx : OFF" ("State")) -> ()  [unwired: 13 in, 6 out]
          }
          frame 4 {
            # "SET Voltage"
            n735 = call "(Sub) CMD Parsing_1.vi"("Set V"=w1137, "State"=(Ctrl)_State_Parcing."Set V") -> ("CMD Set V"=w1136:string, "error out"=w1139:errorcluster)  [unwired: 9 in, 3 out]
            n736 = call "(Instrl) HVPS_1.vi"("Write Data"=w1136, "error in (no error)"=w1139, "CMD"=(Ctrl)_State_HVPS_CMD."Tx : Set V" ("State")) -> ()  [unwired: 11 in, 6 out]
          }
          frame 8 {
            # "SET Current"
            n737 = call "(Sub) CMD Parsing_1.vi"("State"=(Ctrl)_State_Parcing."Set mA", "Set mA"=w1142) -> ("CMD Set mA"=w1141:string, "error out"=w1144:errorcluster)  [unwired: 9 in, 3 out]
            n738 = call "(Instrl) HVPS_1.vi"("Write Data"=w1141, "error in (no error)"=w1144, "CMD"=(Ctrl)_State_HVPS_CMD."Tx : Set mA" ("State")) -> ()  [unwired: 11 in, 6 out]
          }
          frame 16 {
            # "Read Voltage"
            n739 = call "(Instrl) HVPS_1.vi"("CMD"=(Ctrl)_State_HVPS_CMD."Rx : ADC" ("State")) -> ("Get V"=→"G1.Manual_Get V":dbl)  [unwired: 13 in, 5 out]
          }
          frame 32 {
            # "Read Current"
            n740 = call "(Instrl) HVPS_1.vi"("CMD"=(Ctrl)_State_HVPS_CMD."Rx : ADC" ("State")) -> ("Get mA"=→"G1.Manual_Get mA":dbl)  [unwired: 13 in, 5 out]
          }
        }
      }
      event "Group.2 Manual": Value Change {
        n741 = event-data() -> ("NewVal"=w1152:T2)  [unwired: 1 in, 5 out]
        n742 = Unbundle(w1152) -> ("Bool_HV ON"=w1160:bool, "Bool_HV OFF"=w1159:bool, "Bool_Set V"=w1158:bool, "Bool_Set mA"=w1157:bool, "Bool_Get V"=w1156:bool, "Bool_Get mA"=w1155:bool, "Set V"=w1151:u16, "Set mA"=w1150:u16)
        n743 = Build Array(w1160, w1159, w1158, w1157, w1156, w1155) -> (w1154:bool[])
        n744 = Boolean Array To Number(Boolean array=w1154) -> (number=w1153:u32)
        n745 = case shown="8" w1153 {
          tunnel: w1151 -> [_ _ _ w1164 _ _ _]
          tunnel: w1150 -> [_ _ _ _ w1169 _ _]
          frame 0, Default {
          }
          frame 1 {
            # "HV ON"
            n746 = call "(Instrl) HVPS_2.vi"("CMD"=(Ctrl)_State_HVPS_CMD."Tx : ON" ("State")) -> ()  [unwired: 13 in, 6 out]
          }
          frame 2 {
            # "HV OFF"
            n747 = call "(Instrl) HVPS_2.vi"("CMD"=(Ctrl)_State_HVPS_CMD."Tx : OFF" ("State")) -> ()  [unwired: 13 in, 6 out]
          }
          frame 4 {
            # "SET Voltage"
            n748 = call "(Sub) CMD Parsing_2.vi"("Set V"=w1164, "State"=(Ctrl)_State_Parcing."Set V") -> ("CMD Set V"=w1163:string, "error out"=w1166:errorcluster)  [unwired: 9 in, 3 out]
            n749 = call "(Instrl) HVPS_2.vi"("Write Data"=w1163, "error in (no error)"=w1166, "CMD"=(Ctrl)_State_HVPS_CMD."Tx : Set V" ("State")) -> ()  [unwired: 11 in, 6 out]
          }
          frame 8 {
            # "SET Current"
            n750 = call "(Sub) CMD Parsing_2.vi"("State"=(Ctrl)_State_Parcing."Set mA", "Set mA"=w1169) -> ("CMD Set mA"=w1168:string, "error out"=w1171:errorcluster)  [unwired: 9 in, 3 out]
            n751 = call "(Instrl) HVPS_2.vi"("Write Data"=w1168, "error in (no error)"=w1171, "CMD"=(Ctrl)_State_HVPS_CMD."Tx : Set mA" ("State")) -> ()  [unwired: 11 in, 6 out]
          }
          frame 16 {
            # "Read Voltage"
            n752 = call "(Instrl) HVPS_2.vi"("CMD"=(Ctrl)_State_HVPS_CMD."Rx : ADC" ("State")) -> ("Get V"=→"G2.Manual_Get V":dbl)  [unwired: 13 in, 5 out]
          }
          frame 32 {
            # "Read Current"
            n753 = call "(Instrl) HVPS_2.vi"("CMD"=(Ctrl)_State_HVPS_CMD."Rx : ADC" ("State")) -> ("Get mA"=→"G2.Manual_Get mA":dbl)  [unwired: 13 in, 5 out]
          }
        }
      }
      event "Group.3 Manual": Value Change {
        n754 = event-data() -> ("NewVal"=w1179:T2)  [unwired: 1 in, 5 out]
        n755 = Unbundle(w1179) -> ("Bool_HV ON"=w1187:bool, "Bool_HV OFF"=w1186:bool, "Bool_Set V"=w1185:bool, "Bool_Set mA"=w1184:bool, "Bool_Get V"=w1183:bool, "Bool_Get mA"=w1182:bool, "Set V"=w1178:u16, "Set mA"=w1177:u16)
        n756 = Build Array(w1187, w1186, w1185, w1184, w1183, w1182) -> (w1181:bool[])
        n757 = Boolean Array To Number(Boolean array=w1181) -> (number=w1180:u32)
        n758 = case shown="8" w1180 {
          tunnel: w1178 -> [_ _ _ w1191 _ _ _]
          tunnel: w1177 -> [_ _ _ _ w1196 _ _]
          frame 0, Default {
          }
          frame 1 {
            # "HV ON"
            n759 = call "(Instrl) HVPS_3.vi"("CMD"=(Ctrl)_State_HVPS_CMD."Tx : ON" ("State")) -> ()  [unwired: 13 in, 6 out]
          }
          frame 2 {
            # "HV OFF"
            n760 = call "(Instrl) HVPS_3.vi"("CMD"=(Ctrl)_State_HVPS_CMD."Tx : OFF" ("State")) -> ()  [unwired: 13 in, 6 out]
          }
          frame 4 {
            # "SET Voltage"
            n761 = call "(Sub) CMD Parsing_3.vi"("Set V"=w1191, "State"=(Ctrl)_State_Parcing."Set V") -> ("CMD Set V"=w1190:string, "error out"=w1193:errorcluster)  [unwired: 9 in, 3 out]
            n762 = call "(Instrl) HVPS_3.vi"("Write Data"=w1190, "error in (no error)"=w1193, "CMD"=(Ctrl)_State_HVPS_CMD."Tx : Set V" ("State")) -> ()  [unwired: 11 in, 6 out]
          }
          frame 8 {
            # "SET Current"
            n763 = call "(Sub) CMD Parsing_3.vi"("State"=(Ctrl)_State_Parcing."Set mA", "Set mA"=w1196) -> ("CMD Set mA"=w1195:string, "error out"=w1198:errorcluster)  [unwired: 9 in, 3 out]
            n764 = call "(Instrl) HVPS_3.vi"("Write Data"=w1195, "error in (no error)"=w1198, "CMD"=(Ctrl)_State_HVPS_CMD."Tx : Set mA" ("State")) -> ()  [unwired: 11 in, 6 out]
          }
          frame 16 {
            # "Read Voltage"
            n765 = call "(Instrl) HVPS_3.vi"("CMD"=(Ctrl)_State_HVPS_CMD."Rx : ADC" ("State")) -> ("Get V"=→"G3.Manual_Get V":dbl)  [unwired: 13 in, 5 out]
          }
          frame 32 {
            # "Read Current"
            n766 = call "(Instrl) HVPS_3.vi"("CMD"=(Ctrl)_State_HVPS_CMD."Rx : ADC" ("State")) -> ("Get mA"=→"G3.Manual_Get mA":dbl)  [unwired: 13 in, 5 out]
          }
        }
      }
      event "Chamber": Value Change {
        n767 = event-data() -> ("NewVal"=w1204:bool)  [unwired: 1 in, 5 out]
        n768 = case shown="거짓" w1204 {
          frame False {
            n769 = call "(Instrl) Chamber.vi"("State"=(Ctrl)_State_Chamber."Rx : State") -> ("Run ?"=w1205:bool)  [unwired: 7 in, 3 out]
            n770 = case shown="참" w1205 {
              frame False {
              }
              frame True {
                n771 = call "(Instrl) Chamber.vi"("State"=(Ctrl)_State_Chamber."Tx : ON-OFF") -> ()  [unwired: 7 in, 4 out]
              }
            }
          }
          frame True {
            n772 = call "(Instrl) Chamber.vi"("State"=(Ctrl)_State_Chamber."Rx : State") -> ("Run ?"=w1208:bool)  [unwired: 7 in, 3 out]
            n773 = case shown="거짓" w1208 {
              frame False {
                n774 = call "(Instrl) Chamber.vi"("State"=(Ctrl)_State_Chamber."Tx : Target Temp", "Taget Temp"="Target Temp") -> ("error out"=w1211:errorcluster)  [unwired: 6 in, 3 out]
                n775 = call "(Instrl) Chamber.vi"("State"=(Ctrl)_State_Chamber."Tx : ON-OFF", "error in (no error)"=w1211) -> ()  [unwired: 6 in, 4 out]
              }
              frame True {
              }
            }
          }
        }
      }
      event "G1. Start Butten": Value Change {
        n776 = event-data() -> ()  [unwired: 1 in, 6 out]
        n777 = flat-sequence {
          tunnel: w1214 -> [_]
          frame #0 {
            w1215 = FALSE
            n778 = global write "(Var) Get_HVPS_1.vi" "G1. Stop"(w1215) -> ()
            n779 = local write "G1_TEST END?"(FALSE ("G1_TEST END?")) -> ()
            n780 = global write "(Var) Get_HVPS_1.vi" "G1. Q Stop"(w1215) -> ()
          }
          frame #1 {
            n781 = Wait (ms)(milliseconds to wait=u32 100 ("대기 시간 (ms)")) -> ()  [unwired: 1 out]
          }
          frame #2 {
            n782 = global write "(Var) Get_HVPS_1.vi" "G1. Start"(TRUE ("G1. Start")) -> ()
          }
        }
      }
      event "G2. Start Butten": Value Change {
        n783 = event-data() -> ()  [unwired: 1 in, 6 out]
        n784 = flat-sequence {
          tunnel: w1219 -> [_]
          frame #0 {
            w1220 = FALSE
            n785 = global write "(Var) Get_HVPS_2.vi" "G2. Stop"(w1220) -> ()
            n786 = global write "(Var) Get_HVPS_2.vi" "G2. Q Stop"(w1220) -> ()
            n787 = local write "G2_TEST END?"(FALSE ("G1_TEST END?")) -> ()
          }
          frame #1 {
            n788 = Wait (ms)(milliseconds to wait=u32 100 ("대기 시간 (ms)")) -> ()  [unwired: 1 out]
          }
          frame #2 {
            n789 = global write "(Var) Get_HVPS_2.vi" "G2. Start"(TRUE) -> ()
          }
        }
      }
      event "G3. Start Butten": Value Change {
        n790 = event-data() -> ()  [unwired: 1 in, 6 out]
        n791 = flat-sequence {
          tunnel: w1224 -> [_]
          frame #0 {
            w1225 = FALSE
            n792 = global write "(Var) Get_HVPS_3.vi" "G3. Stop"(w1225) -> ()
            n793 = global write "(Var) Get_HVPS_3.vi" "G3. Q Stop"(w1225) -> ()
            n794 = local write "G3_TEST END?"(FALSE ("G1_TEST END?")) -> ()
          }
          frame #1 {
            n795 = Wait (ms)(milliseconds to wait=u32 100 ("대기 시간 (ms)")) -> ()  [unwired: 1 out]
          }
          frame #2 {
            n796 = global write "(Var) Get_HVPS_3.vi" "G3. Start"(TRUE) -> ()
          }
        }
      }
      event "G1. Stop Butten": Value Change {
        n797 = event-data() -> ()  [unwired: 1 in, 6 out]
        n798 = flat-sequence {
          tunnel: w1229 -> [_]
          frame #0 {
            n799 = global write "(Var) Get_HVPS_1.vi" "G1. Start"(FALSE ("G1. Start")) -> ()
          }
          frame #1 {
            n800 = Wait (ms)(milliseconds to wait=u32 100 ("대기 시간 (ms)")) -> ()  [unwired: 1 out]
          }
          frame #2 {
            n801 = global write "(Var) Get_HVPS_1.vi" "G1. Stop"(TRUE) -> ()
          }
        }
      }
      event "G2. Stop Butten": Value Change {
        n802 = event-data() -> ()  [unwired: 1 in, 6 out]
        n803 = flat-sequence {
          tunnel: w1233 -> [_]
          frame #0 {
            n804 = global write "(Var) Get_HVPS_2.vi" "G2. Start"(FALSE ("G2. Start")) -> ()
          }
          frame #1 {
            n805 = Wait (ms)(milliseconds to wait=u32 100 ("대기 시간 (ms)")) -> ()  [unwired: 1 out]
          }
          frame #2 {
            n806 = global write "(Var) Get_HVPS_2.vi" "G2. Stop"(TRUE) -> ()
          }
        }
      }
      event "G3. Stop Butten": Value Change {
        n807 = event-data() -> ()  [unwired: 1 in, 6 out]
        n808 = flat-sequence {
          tunnel: w1237 -> [_]
          frame #0 {
            n809 = global write "(Var) Get_HVPS_3.vi" "G3. Start"(FALSE) -> ()
          }
          frame #1 {
            n810 = Wait (ms)(milliseconds to wait=u32 100 ("대기 시간 (ms)")) -> ()  [unwired: 1 out]
          }
          frame #2 {
            n811 = global write "(Var) Get_HVPS_3.vi" "G3. Stop"(TRUE) -> ()
          }
        }
      }
      event "G1. RB/GB": Value Change {
        n812 = event-data() -> ("NewVal"=w1241:bool)  [unwired: 1 in, 5 out]
        n813 = case shown="참" w1241 {
          frame True {
            # "GB"
            n814 = local write "G1. Taget Voltage"(0.0 ("G1. Taget Voltage")) -> ()
            n815 = property on="G1. Taget Voltage" class="DigNum (엄격한)"("Maximum"=30.0 ("데이터 입력 제한:최대")) -> ()  [unwired: 2 in, 2 out]
            n816 = local write "G1. Layout"(TRUE) -> ()
          }
          frame False {
            # "RB"
            n817 = local write "G1. Taget Voltage"(0.0 ("G1. Taget Voltage")) -> ()
            n818 = property on="G1. Taget Voltage" class="DigNum (엄격한)"("Maximum"=2000.0 ("데이터 입력 제한:최대")) -> ()  [unwired: 2 in, 2 out]
            n819 = local write "G1. Layout"(FALSE) -> ()
          }
        }
      }
      event "G2. RB/GB": Value Change {
        n820 = event-data() -> ("NewVal"=w1248:bool)  [unwired: 1 in, 5 out]
        n821 = case shown="참" w1248 {
          frame True {
            # "GB"
            n822 = local write "G2. Taget Voltage"(0.0 ("G1. Taget Voltage")) -> ()
            n823 = property on="G2. Taget Voltage" class="DigNum (엄격한)"("Maximum"=30.0 ("데이터 입력 제한:최대")) -> ()  [unwired: 2 in, 2 out]
            n824 = local write "G2. Layout"(TRUE) -> ()
          }
          frame False {
            # "RB"
            n825 = local write "G2. Taget Voltage"(0.0 ("G1. Taget Voltage")) -> ()
            n826 = property on="G2. Taget Voltage" class="DigNum (엄격한)"("Maximum"=2000.0 ("데이터 입력 제한:최대")) -> ()  [unwired: 2 in, 2 out]
            n827 = local write "G2. Layout"(FALSE) -> ()
          }
        }
      }
      event "G3. RB/GB": Value Change {
        n828 = event-data() -> ("NewVal"=w1255:bool)  [unwired: 1 in, 5 out]
        n829 = case shown="참" w1255 {
          frame True {
            # "GB"
            n830 = local write "G3. Taget Voltage"(0.0 ("G1. Taget Voltage")) -> ()
            n831 = property on="G3. Taget Voltage" class="DigNum (엄격한)"("Maximum"=30.0 ("데이터 입력 제한:최대")) -> ()  [unwired: 2 in, 2 out]
            n832 = local write "G3. Layout"(TRUE) -> ()
          }
          frame False {
            # "RB"
            n833 = local write "G3. Taget Voltage"(0.0 ("G1. Taget Voltage")) -> ()
            n834 = property on="G3. Taget Voltage" class="DigNum (엄격한)"("Maximum"=2000.0 ("데이터 입력 제한:최대")) -> ()  [unwired: 2 in, 2 out]
            n835 = local write "G3. Layout"(FALSE) -> ()
          }
        }
      }
      event "Exit": Value Change {
        n836 = event-data() -> ()  [unwired: 1 in, 1 out]
        n837 = Two Button Dialog(message="프로그램을 종료하시겠습니까?" ("메시지")) -> (T button?=w1264:bool)  [unwired: 2 in]
        n838 = case shown="참" w1264 {
          tunnel: [FALSE TRUE] -> w1263
          frame False {
          }
          frame True {
            w1268 = TRUE ("Quick Stop")
            w1269 = FALSE ("Test Start ?")
            w1267 = TRUE ("Quick Stop")
            n839 = global write "(Var) Get_HVPS_1.vi" "G1. Q Stop"(w1267) -> ()
            n840 = global write "(Var) Get_HVPS_2.vi" "G2. Q Stop"(w1267) -> ()
            n841 = global write "(Var) Get_HVPS_3.vi" "G3. Q Stop"(w1267) -> ()
            n842 = global write "(Var) Get_HVPS_1.vi" "G1. Stop"(w1268) -> ()
            n843 = global write "(Var) Get_HVPS_2.vi" "G2. Stop"(w1268) -> ()
            n844 = global write "(Var) Get_HVPS_3.vi" "G3. Stop"(w1268) -> ()
            n845 = global write "(Var) Get_HVPS_1.vi" "G1. Start"(w1269) -> ()
            n846 = global write "(Var) Get_HVPS_2.vi" "G2. Start"(w1269) -> ()
            n847 = global write "(Var) Get_HVPS_3.vi" "G3. Start"(w1269) -> ()
          }
        }
        "Exit ?" <- w1263
      }
      event Panel Close? {
        n848 = event-data() -> ()  [unwired: 1 in, 4 out]
        n849 = Two Button Dialog(message="프로그램을 종료하시겠습니까?" ("메시지")) -> (T button?=w1274:bool)  [unwired: 2 in]
        n850 = case shown="참" w1274 {
          tunnel: [FALSE TRUE] -> w1271
          frame False {
          }
          frame True {
            w1278 = TRUE ("Quick Stop")
            w1279 = FALSE ("Test Start ?")
            w1277 = TRUE ("Quick Stop")
            n851 = global write "(Var) Get_HVPS_1.vi" "G1. Q Stop"(w1277) -> ()
            n852 = global write "(Var) Get_HVPS_2.vi" "G2. Q Stop"(w1277) -> ()
            n853 = global write "(Var) Get_HVPS_1.vi" "G1. Stop"(w1278) -> ()
            n854 = global write "(Var) Get_HVPS_2.vi" "G2. Stop"(w1278) -> ()
            n855 = global write "(Var) Get_HVPS_3.vi" "G3. Q Stop"(w1277) -> ()
            n856 = global write "(Var) Get_HVPS_3.vi" "G3. Stop"(w1278) -> ()
            n857 = global write "(Var) Get_HVPS_1.vi" "G1. Start"(w1279) -> ()
            n858 = global write "(Var) Get_HVPS_2.vi" "G2. Start"(w1279) -> ()
            n859 = global write "(Var) Get_HVPS_3.vi" "G3. Start"(w1279) -> ()
          }
        }
        n860 = local write "Exit ?"(w1271) -> ()
        n861 = event-data("Discard?"=TRUE ("버림?")) -> ()  [unwired: 1 in, 1 out]
      }
    }
  }
  n862 = Merge Errors(w19, w17, w6, w8) -> (w4:errorcluster)
  n863 = flat-sequence {
    tunnel: w4 -> [w1282]
    tunnel: [w1282] -> w3
    frame #0 {
      "END" <- TRUE
    }
  }
  n864 = Merge Errors(w3, w10) -> (w11:errorcluster)
  n865 = property class="App"(error in=w11) -> (error out=w20:errorcluster, "App.Kind"=w21:T12)  [unwired: 1 in, 1 out]
  n866 = case shown="\"Run Time System\"" w21 {
    tunnel: w20 -> [_ _ w1284 _ _ _ _]
    tunnel: [_ _ w1284 _ _ _ _] -> w18
    frame "invalid app kind", Default {
    }
    frame "Development System" {
    }
    frame "Run Time System" {
      n867 = Quit LabVIEW(quit? (T)=TRUE ("종료? (참)")) -> ()
    }
    frame "Student Edition" {
    }
    frame "Embedded LabVIEW" {
    }
    frame "Evaluation" {
    }
    frame "Custom" {
    }
  }
  "error out" <- w18
